vi "总磷总氮通讯.vi"() -> ()   [LabVIEW 2016, in "斯坦道氨氮.lvlib"]
uses:
  <vilib>/Utility/config.llb/NI_LVConfig.lvlib
  <vilib>/Plasmionique/MB Master/MB_Master/MB_Master.lvclass
  <vilib>/Plasmionique/MB Master/MB Master.lvlib
  <vilib>/ptbypt/NI_PtbyPt.lvlib
  <vilib>/Plasmionique/MB Master/MB_Master_Serial/MB_Master_Serial.lvclass
  <vilib>/Plasmionique/MB Master/MB_Master_TCP/MB_Master_TCP.lvclass
  <vilib>/Utility/config.llb/Write Key (Boolean).vi
  <vilib>/Utility/config.llb/Write Key (String).vi
  C:/Program Files (x86)/National Instruments/LabVIEW 2016/vi.lib/Plasmionique/MB Master/MB_Master/MB_Master.lvclass
panel:
  out "启用":bool=TRUE
  out "氨氮状态告警区":u16[](array[numeric])
  out "氨氮测量数据区":u16[](array[numeric])
  out "COD测量数据区":u16[](array[numeric])
  out "COD状态告警区":u16[](array[numeric])
  out "总氮测量数据区":u16[](array[numeric])
  out "总氮状态告警区":u16[](array[numeric])
  out "总磷状态告警区":u16[](array[numeric])
  out "总磷测量数据区":u16[](array[numeric])
  out "状态告警区":T1 {"告警代码" items=["无告警", "缺试剂告警", "缺水样告警", "缺蒸馏水告警", "缺标液告警", "仪表漏液告警", "标定异常告警", "超量程告警", "加热异常", "低试剂预警", "超上限告警", "超下限告警", "仪表内部其他异常", "滴定异常告警", "电极异常告警", "量程切换告警", "参数设置告警", "PH电极电位异常", "电导率电极异常", "浊度光度异常", "溶解氧电极异常", "溶解氧光强异常", "温度异常告警", "PH异常告警", "溶解氧异常告警", "电导率异常告警", "浊度异常告警", "叶绿素异常告警", "藻密度异常告警", "蓝绿藻异常告警", "ORP异常告警", "氨氮异常告警", "清洁刷异常告警", "SD卡异常告警", "蓝牙异常告警", "Wifi异常告警", "流程异常告警"]; "故障代码" items=["无故障", "电机故障", "温度故障", "通讯故障", "滴定故障"]}
  out "测量数据区":T2 {"单位" items=["ug/L", "mg/L", "ppm", "mg/m3", "cm", "ppb", "ug/m3", "%", "nmol/mol", "umol/mol", "MPN/L", "MPN/100ml", "ng/m3", "NTU", "无量纲", "ms/cm", "us/cm", "℃", "mV", "万个/L"]}
  out "status":bool
  out "关键参数区":T3
  in  "读关键参数区":bool
  in  "读状态告警区":bool
  in  "读测量数据区":bool
  in  "站号":u16(ring) items=["总磷"=1, "氨氮"=3]
  in  "停止":bool
  in  "启动":bool
  in  "控制命令":u16(ring) items=["启动测量"=1, "标样核查"=2, "零点核查"=3, "跨度核查"=4, "空白测试"=5, "平行样测试"=6, "加标回收"=7, "空白校准"=8, "标样校准"=9, "初始化（清洗）"=10, "停止测试"=11, "仪器重启"=12, "校时"=13, "模式设置"=14, "测量间隔设置"=15]
  in  "控制命令参数":u16[](array[numeric]) format="%04xH"
  in  "VISA Resource":refnum<visa-resource-name>
  in  "启用模块":bool
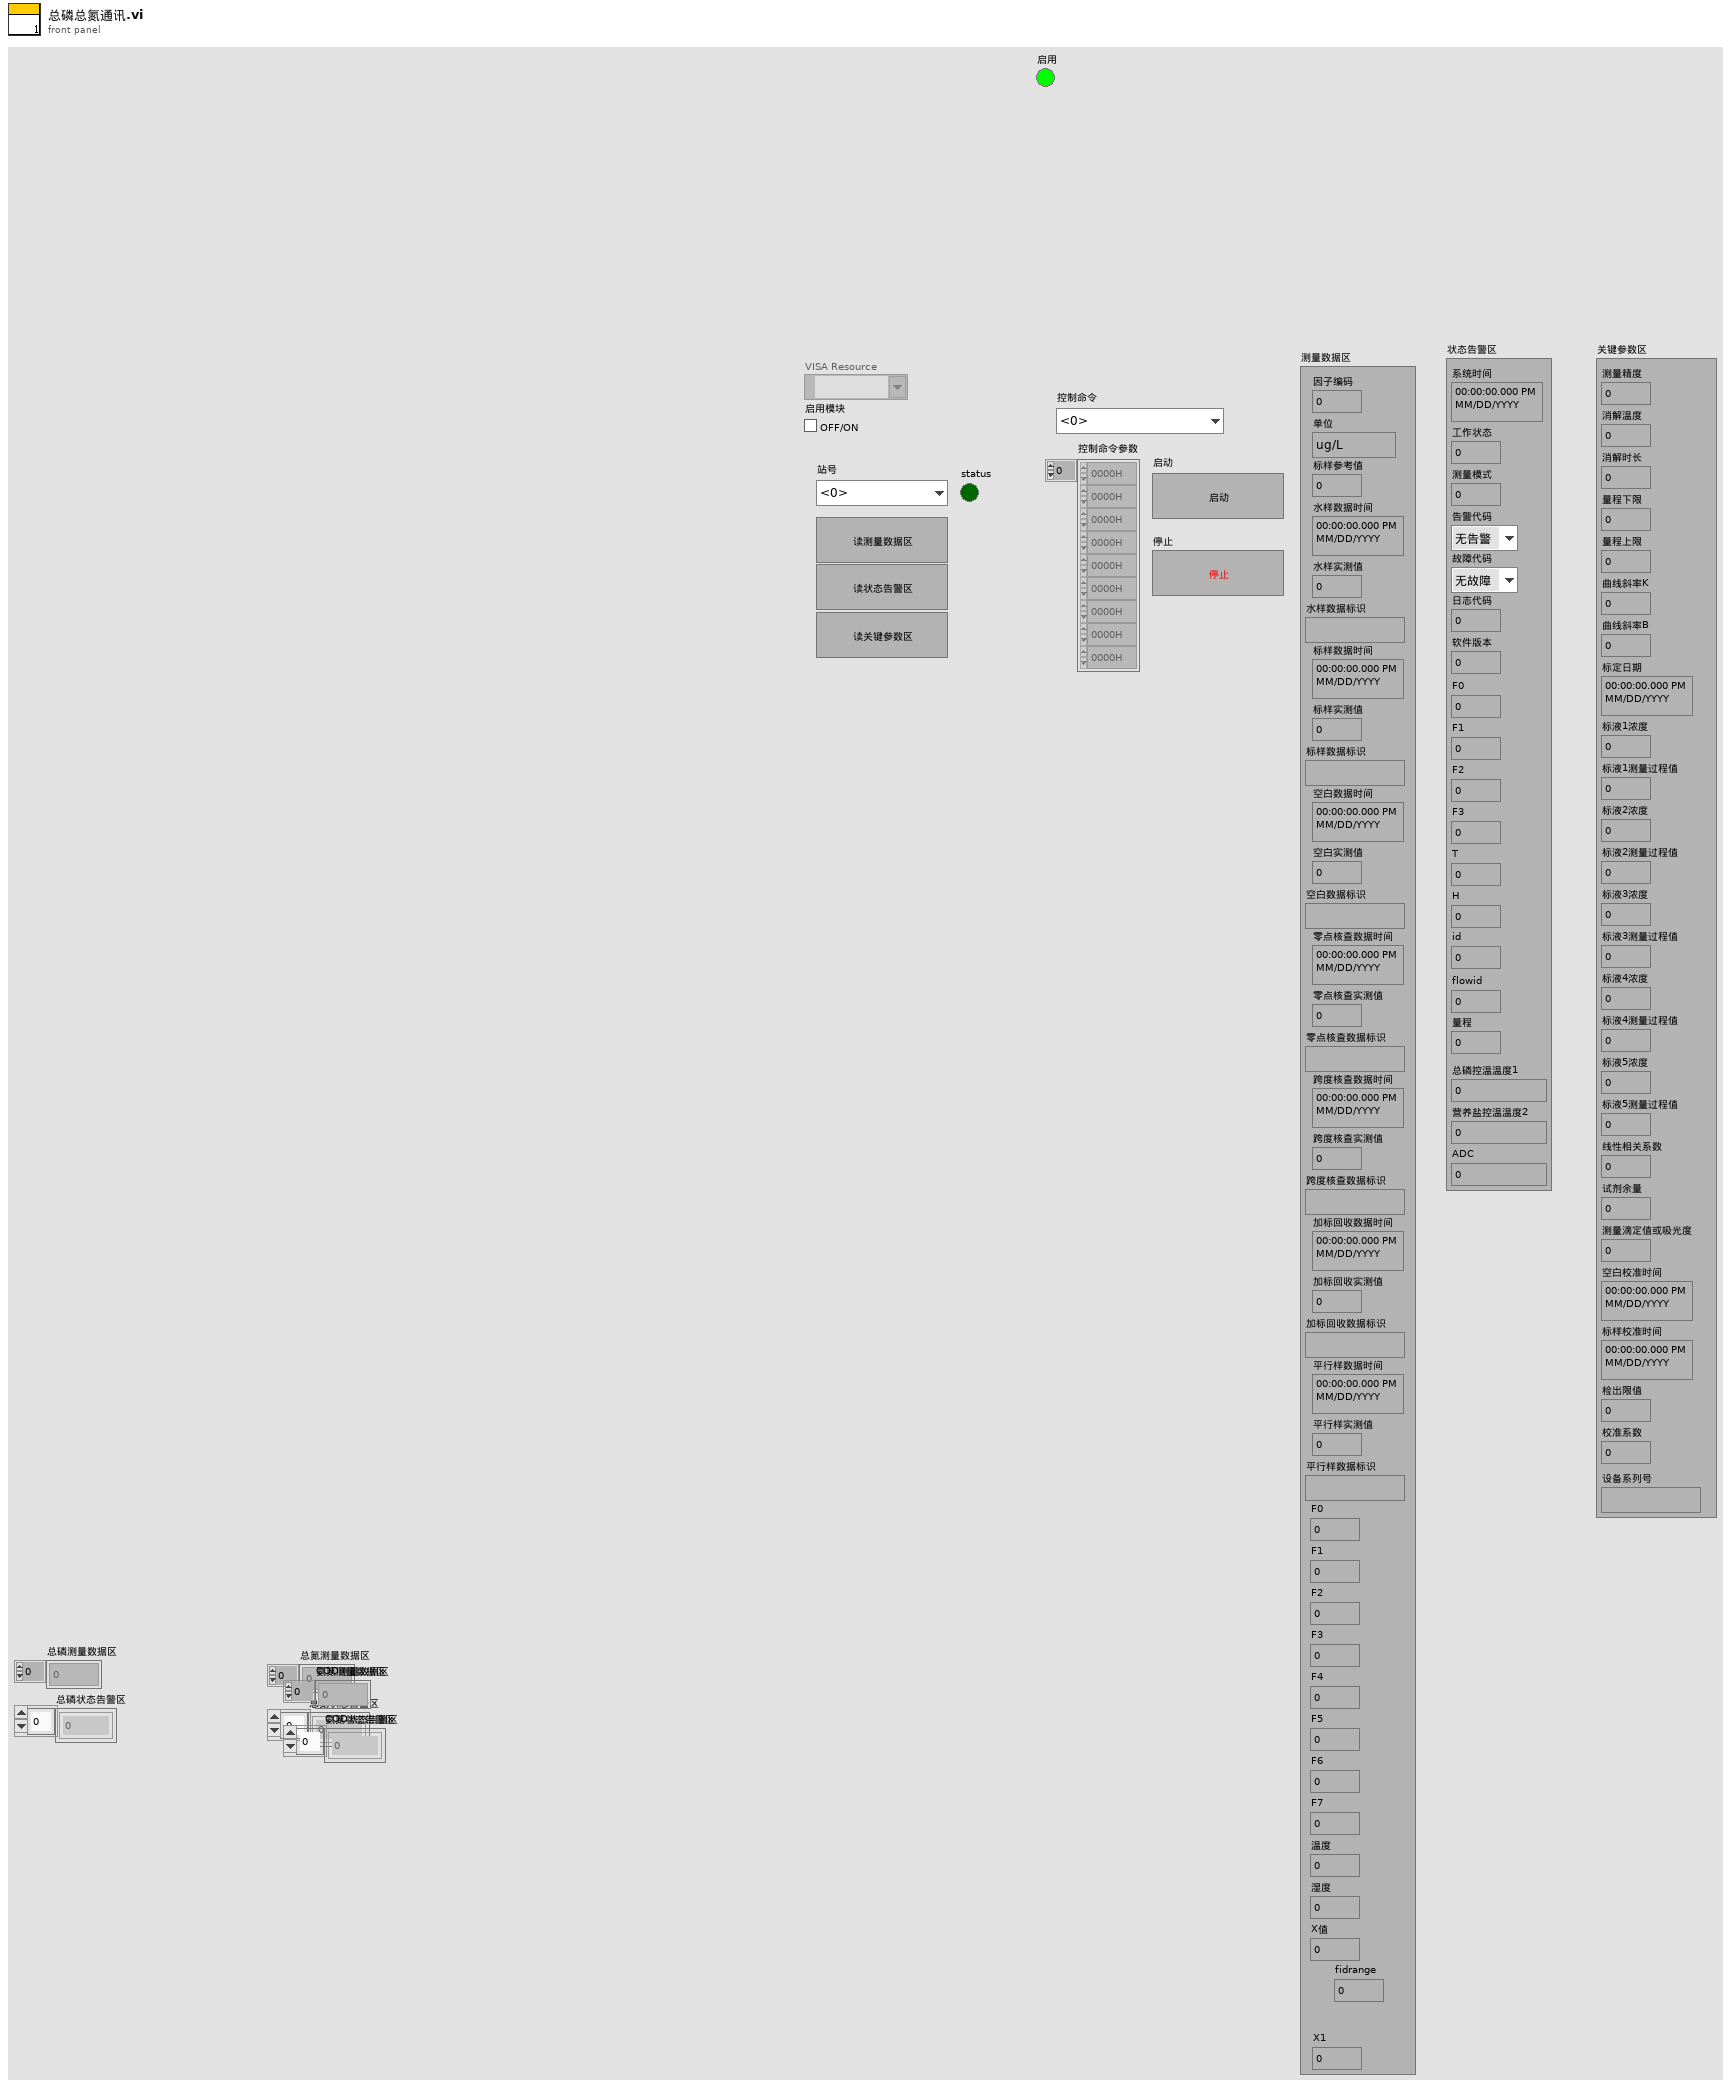
[diagram p1: front panel]
types:
  T1 = cluster{"系统时间":timestamp, "工作状态":u16, "测量模式":u16, "告警代码":u16, "故障代码":u16, "日志代码":u16, "软件版本":u16, "F0":sgl, "F1":sgl, "F2":sgl, "F3":sgl, "T":sgl, "H":sgl, "id":u16, "flowid":u16, "量程":u16, "总磷控温温度1":sgl, "营养盐控温温度2":sgl, "ADC":sgl}
  T2 = cluster{"因子编码":u32, "单位":u16, "标样参考值":sgl, "水样数据时间":timestamp, "水样实测值":sgl, "水样数据标识":string, "标样数据时间":timestamp, "标样实测值":sgl, "标样数据标识":string, "空白数据时间":timestamp, "空白实测值":sgl, "空白数据标识":string, "零点核查数据时间":timestamp, "零点核查实测值":sgl, "零点核查数据标识":string, "跨度核查数据时间":timestamp, "跨度核查实测值":sgl, "跨度核查数据标识":string, "加标回收数据时间":timestamp, "加标回收实测值":sgl, "加标回收数据标识":string, "平行样数据时间":timestamp, "平行样实测值":sgl, "平行样数据标识":string, "F0":sgl, "F1":sgl, "F2":sgl, "F3":sgl, "F4":sgl, "F5":sgl, "F6":sgl, "F7":sgl, "温度":sgl, "湿度":sgl, "X值":sgl, "fidrange":u16, "X1":sgl}
  T3 = cluster{"测量精度":u16, "消解温度":u16, "消解时长":u16, "量程下限":sgl, "量程上限":sgl, "曲线斜率K":sgl, "曲线斜率B":sgl, "标定日期":timestamp, "标液1浓度":sgl, "标液1测量过程值":sgl, "标液2浓度":sgl, "标液2测量过程值":sgl, "标液3浓度":sgl, "标液3测量过程值":sgl, "标液4浓度":sgl, "标液4测量过程值":sgl, "标液5浓度":sgl, "标液5测量过程值":sgl, "线性相关系数":sgl, "试剂余量":u32, "测量滴定值或吸光度":sgl, "空白校准时间":timestamp, "标样校准时间":timestamp, "检出限值":sgl, "校准系数":sgl, "设备系列号":string}
  T4 = cluster{"系统时间":timestamp, "工作状态":u16, "测量模式":enum16{"待机", "连续模式", "周期模式", "定点模式", "受控模式", "手动模式"}, "告警代码":u16, "故障代码":u16, "日志代码":u16, "软件版本":u16, "F0":sgl, "F1":sgl, "F2":sgl, "F3":sgl, "T":sgl, "H":sgl, "id":u16, "flowid":u16, "量程":u16, "总磷控温温度1":sgl, "营养盐控温温度2":sgl, "ADC":sgl}
  T5 = cluster{"因子编码":u32, "单位":u16, "标样参考值":sgl, "水样数据时间":timestamp, "水样实测值":sgl, "水样数据标识":string, "标样数据时间":timestamp, "标样实测值":sgl, "标样数据标识":string, "空白数据时间":timestamp, "空白实测值":sgl, "空白数据标识":string, "零点核查数据时间":timestamp, "零点核查实测值":sgl, "零点核查数据标识":string, "跨度核查数据时间":timestamp, "跨度核查实测值":sgl, "跨度核查数据标识":string, "加标回收数据时间":timestamp, "加标回收实测值":sgl, "加标回收数据标识":string, "平行样数据时间":timestamp, "平行样实测值":sgl, "平行样数据标识":string, "F0":sgl, "F1":sgl, "F2":sgl, "F3":sgl, "F4":sgl, "F5":sgl, "F6":sgl, "F7":sgl, "温度":sgl, "湿度":sgl, "X值":sgl, "fidrange":u16, "X1值":sgl}
  T6 = cluster{"测量精度":u16, "消解温度":u16, "消解时长":u16, "量程下限":sgl, "量程上限":sgl, "曲线斜率K":sgl, "曲线斜率B":sgl, "标定日期":timestamp, "标液1浓度":sgl, "标液1测量过程值":sgl, "标液2浓度":sgl, "标液2测量过程值":sgl, "标液3浓度":sgl, "标液3测量过程值":sgl, "标液4浓度":sgl, "标液4测量过程值":sgl, "标液5浓度":sgl, "标液5测量过程值":sgl, "线性相关系数":sgl, "试剂余量":u32, "测量滴定值或吸光度":sgl, "空白校准时间":timestamp, "标样校准时间":timestamp, "检出限值":sgl, "校准系数":sgl, "设备系列号":string}[]
  T7 = cluster{"系统时间":timestamp, "工作状态":u16, "测量模式":enum16{"待机", "连续模式", "周期模式", "定点模式", "受控模式", "手动模式"}, "告警代码":u16, "故障代码":u16, "日志代码":u16, "软件版本":u16, "F0":sgl, "F1":sgl, "F2":sgl, "F3":sgl, "T":sgl, "H":sgl, "id":u16, "flowid":u16, "量程":u16, "总磷控温温度1":sgl, "营养盐控温温度2":sgl, "ADC":sgl}[]
  T8 = cluster{"因子编码":u32, "单位":u16, "标样参考值":sgl, "水样数据时间":timestamp, "水样实测值":sgl, "水样数据标识":string, "标样数据时间":timestamp, "标样实测值":sgl, "标样数据标识":string, "空白数据时间":timestamp, "空白实测值":sgl, "空白数据标识":string, "零点核查数据时间":timestamp, "零点核查实测值":sgl, "零点核查数据标识":string, "跨度核查数据时间":timestamp, "跨度核查实测值":sgl, "跨度核查数据标识":string, "加标回收数据时间":timestamp, "加标回收实测值":sgl, "加标回收数据标识":string, "平行样数据时间":timestamp, "平行样实测值":sgl, "平行样数据标识":string, "F0":sgl, "F1":sgl, "F2":sgl, "F3":sgl, "F4":sgl, "F5":sgl, "F6":sgl, "F7":sgl, "温度":sgl, "湿度":sgl, "X值":sgl, "fidrange":u16, "X1值":sgl}[]
  T9 = typedef "CODCr交互.ctl" = cluster{"状态告警区":cluster{"系统时间":timestamp, "工作状态":u16, "测量模式":enum16{"待机", "连续模式", "周期模式", "定点模式", "受控模式", "手动模式"}, "告警代码":u16, "故障代码":u16, "日志代码":u16, "软件版本":u16, "F0":sgl, "F1":sgl, "F2":sgl, "F3":sgl, "T":sgl, "H":sgl, "id":u16, "flowid":u16, "量程":u16, "总磷控温温度1":sgl, "营养盐控温温度2":sgl, "ADC":sgl}, "平台试剂余量百分比":sgl, "关键参数":cluster{"测量量程":dbl, "测量精度":dbl, "测量间隔":dbl, "消解温度":dbl, "消解时长":dbl, "空白校准时间":timestamp, "曲线截距":dbl, "曲线斜率":dbl, "测量检出限":dbl, "测量信号值":dbl, "线性相关系数":dbl, "二次多项式系数":dbl, "标样校准时间":timestamp, "稀释倍数":dbl, "三项式系数":dbl, "空白标定系数":dbl, "量程系数":dbl, "F0/ORPA":dbl, "F1/ORPB":dbl, "F2/ORPK":dbl, "F3":dbl, "F4":dbl, "F5":dbl, "F6":dbl, "F7":dbl, "X0/滴定数":dbl, "量程":dbl}, "关键参数改变":bool, "校准信息":cluster{"低标液1浓度":dbl, "低标液1信号值":dbl, "低标液1启用":u16, "低标液2浓度":dbl, "低标液2信号值":dbl, "低标液2启用":u16, "低标液3浓度":dbl, "低标液3信号值":dbl, "低标液3启用":u16, "低标液4浓度":dbl, "低标液4信号值":dbl, "低标液4启用":u16, "低标液5浓度":dbl, "低标液5信号值":dbl, "低标液5启用":u16, "高标液1浓度":dbl, "高标液1信号值":dbl, "高标液1启用":u16, "高标液2浓度":dbl, "高标液2信号值":dbl, "高标液2启用":u16, "高标液3浓度":dbl, "高标液3信号值":dbl, "高标液3启用":u16, "高标液4浓度":dbl, "高标液4信号值":dbl, "高标液4启用":u16, "高标液5浓度":dbl, "高标液5信号值":dbl, "高标液5启用":u16}, "校准信息改变":bool}
  T10 = typedef "总磷交互.ctl" = cluster{"状态告警区":cluster{"系统时间":timestamp, "工作状态":u16, "测量模式":enum16{"待机", "连续模式", "周期模式", "定点模式", "受控模式", "手动模式"}, "告警代码":u16, "故障代码":u16, "日志代码":u16, "软件版本":u16, "F0":sgl, "F1":sgl, "F2":sgl, "F3":sgl, "T":sgl, "H":sgl, "id":u16, "flowid":u16, "量程":u16, "总磷控温温度1":sgl, "营养盐控温温度2":sgl, "ADC":sgl}, "平台试剂余量百分比":sgl, "关键参数":cluster{"测量量程":dbl, "测量精度":dbl, "测量间隔":dbl, "消解温度":dbl, "消解时长":dbl, "空白校准时间":timestamp, "曲线截距":dbl, "曲线斜率":dbl, "测量检出限":dbl, "测量信号值":dbl, "线性相关系数":dbl, "二次多项式系数":dbl, "标样校准时间":timestamp, "稀释倍数":dbl, "三项式系数":dbl, "空白标定系数":dbl, "量程系数":dbl, "F0/ORPA":dbl, "F1/ORPB":dbl, "F2/ORPK":dbl, "F3":dbl, "F4":dbl, "F5":dbl, "F6":dbl, "F7":dbl, "X0/滴定数":dbl, "量程":dbl}, "关键参数改变":bool, "校准信息":cluster{"低标液1浓度":dbl, "低标液1信号值":dbl, "低标液1启用":u16, "低标液2浓度":dbl, "低标液2信号值":dbl, "低标液2启用":u16, "低标液3浓度":dbl, "低标液3信号值":dbl, "低标液3启用":u16, "低标液4浓度":dbl, "低标液4信号值":dbl, "低标液4启用":u16, "低标液5浓度":dbl, "低标液5信号值":dbl, "低标液5启用":u16, "高标液1浓度":dbl, "高标液1信号值":dbl, "高标液1启用":u16, "高标液2浓度":dbl, "高标液2信号值":dbl, "高标液2启用":u16, "高标液3浓度":dbl, "高标液3信号值":dbl, "高标液3启用":u16, "高标液4浓度":dbl, "高标液4信号值":dbl, "高标液4启用":u16, "高标液5浓度":dbl, "高标液5信号值":dbl, "高标液5启用":u16}, "校准信息改变":bool}
  T11 = typedef "总氮交互.ctl" = cluster{"状态告警区":cluster{"系统时间":timestamp, "工作状态":u16, "测量模式":enum16{"待机", "连续模式", "周期模式", "定点模式", "受控模式", "手动模式"}, "告警代码":u16, "故障代码":u16, "日志代码":u16, "软件版本":u16, "F0":sgl, "F1":sgl, "F2":sgl, "F3":sgl, "T":sgl, "H":sgl, "id":u16, "flowid":u16, "量程":u16, "总磷控温温度1":sgl, "营养盐控温温度2":sgl, "ADC":sgl}, "平台试剂余量百分比":sgl, "关键参数":cluster{"测量量程":dbl, "测量精度":dbl, "测量间隔":dbl, "消解温度":dbl, "消解时长":dbl, "空白校准时间":timestamp, "曲线截距":dbl, "曲线斜率":dbl, "测量检出限":dbl, "测量信号值":dbl, "线性相关系数":dbl, "二次多项式系数":dbl, "标样校准时间":timestamp, "稀释倍数":dbl, "三项式系数":dbl, "空白标定系数":dbl, "量程系数":dbl, "F0/ORPA":dbl, "F1/ORPB":dbl, "F2/ORPK":dbl, "F3":dbl, "F4":dbl, "F5":dbl, "F6":dbl, "F7":dbl, "X0/滴定数":dbl, "量程":dbl}, "关键参数改变":bool, "校准信息":cluster{"低标液1浓度":dbl, "低标液1信号值":dbl, "低标液1启用":u16, "低标液2浓度":dbl, "低标液2信号值":dbl, "低标液2启用":u16, "低标液3浓度":dbl, "低标液3信号值":dbl, "低标液3启用":u16, "低标液4浓度":dbl, "低标液4信号值":dbl, "低标液4启用":u16, "低标液5浓度":dbl, "低标液5信号值":dbl, "低标液5启用":u16, "高标液1浓度":dbl, "高标液1信号值":dbl, "高标液1启用":u16, "高标液2浓度":dbl, "高标液2信号值":dbl, "高标液2启用":u16, "高标液3浓度":dbl, "高标液3信号值":dbl, "高标液3启用":u16, "高标液4浓度":dbl, "高标液4信号值":dbl, "高标液4启用":u16, "高标液5浓度":dbl, "高标液5信号值":dbl, "高标液5启用":u16}, "校准信息改变":bool}
  T12 = typedef "氨氮交互.ctl" = cluster{"状态告警区":cluster{"系统时间":timestamp, "工作状态":u16, "测量模式":enum16{"待机", "连续模式", "周期模式", "定点模式", "受控模式", "手动模式"}, "告警代码":u16, "故障代码":u16, "日志代码":u16, "软件版本":u16, "F0":sgl, "F1":sgl, "F2":sgl, "F3":sgl, "T":sgl, "H":sgl, "id":u16, "flowid":u16, "量程":u16, "总磷控温温度1":sgl, "营养盐控温温度2":sgl, "ADC":sgl}, "平台试剂余量百分比":sgl, "关键参数":cluster{"测量量程":dbl, "测量精度":dbl, "测量间隔":dbl, "消解温度":dbl, "消解时长":dbl, "空白校准时间":timestamp, "曲线截距":dbl, "曲线斜率":dbl, "测量检出限":dbl, "测量信号值":dbl, "线性相关系数":dbl, "二次多项式系数":dbl, "标样校准时间":timestamp, "稀释倍数":dbl, "三项式系数":dbl, "空白标定系数":dbl, "量程系数":dbl, "F0/ORPA":dbl, "F1/ORPB":dbl, "F2/ORPK":dbl, "F3":dbl, "F4":dbl, "F5":dbl, "F6":dbl, "F7":dbl, "X0/滴定数":dbl, "量程":dbl}, "关键参数改变":bool, "校准信息":cluster{"低标液1浓度":dbl, "低标液1信号值":dbl, "低标液1启用":u16, "低标液2浓度":dbl, "低标液2信号值":dbl, "低标液2启用":u16, "低标液3浓度":dbl, "低标液3信号值":dbl, "低标液3启用":u16, "低标液4浓度":dbl, "低标液4信号值":dbl, "低标液4启用":u16, "低标液5浓度":dbl, "低标液5信号值":dbl, "低标液5启用":u16, "高标液1浓度":dbl, "高标液1信号值":dbl, "高标液1启用":u16, "高标液2浓度":dbl, "高标液2信号值":dbl, "高标液2启用":u16, "高标液3浓度":dbl, "高标液3信号值":dbl, "高标液3启用":u16, "高标液4浓度":dbl, "高标液4信号值":dbl, "高标液4启用":u16, "高标液5浓度":dbl, "高标液5信号值":dbl, "高标液5启用":u16}, "校准信息改变":bool}
  T13 = typedef "NI_LVConfig.lvlib/Config Data RefNum.ctl" = refnum<k1>
  T14 = enum8{"Enabled", "Disabled", "Disabled and Grayed Out"}
  T15 = typedef "报警信息字段定义.ctl" = cluster{"时间":timestamp, "参数":string, "报警信息":string, "备注":string, "code":u64, "platform_alarm_code":string, "报警标识":enum16{"产生", "消除"}}
  T16 = cluster{"baud rate (bps)":u32, "stop bits":u16, "parity":u16, "flow control":u16, "timeout":u32, "retries":i32}
  T17 = cluster{"测量量程":dbl, "测量精度":dbl, "测量间隔":dbl, "消解温度":dbl, "消解时长":dbl, "空白校准时间":timestamp, "曲线截距":dbl, "曲线斜率":dbl, "测量检出限":dbl, "测量信号值":dbl, "线性相关系数":dbl, "二次多项式系数":dbl, "标样校准时间":timestamp, "稀释倍数":dbl, "三项式系数":dbl, "空白标定系数":dbl, "量程系数":dbl, "F0/ORPA":dbl, "F1/ORPB":dbl, "F2/ORPK":dbl, "F3":dbl, "F4":dbl, "F5":dbl, "F6":dbl, "F7":dbl, "X0/滴定数":dbl, "量程":dbl}
  T18 = typedef "斯坦道氨氮.lvlib/关键参数.ctl" = cluster{"测量量程":sgl, "测量检出限":sgl, "测量精度":sgl, "测量间隔":sgl, "消解温度":sgl, "消解时长":sgl, "三项式系数":sgl, "二次多项式系数":sgl, "曲线斜率":sgl, "曲线截距":sgl, "线性相关系数":sgl, "空白校准时间":timestamp, "标样校准时间":timestamp, "测量信号值":sgl, "稀释倍数":sgl, "空白标定系数":sgl, "量程系数":sgl}
  T19 = cluster{"低标液1浓度":dbl, "低标液1信号值":dbl, "低标液1启用":u16, "低标液2浓度":dbl, "低标液2信号值":dbl, "低标液2启用":u16, "低标液3浓度":dbl, "低标液3信号值":dbl, "低标液3启用":u16, "低标液4浓度":dbl, "低标液4信号值":dbl, "低标液4启用":u16, "低标液5浓度":dbl, "低标液5信号值":dbl, "低标液5启用":u16, "高标液1浓度":dbl, "高标液1信号值":dbl, "高标液1启用":u16, "高标液2浓度":dbl, "高标液2信号值":dbl, "高标液2启用":u16, "高标液3浓度":dbl, "高标液3信号值":dbl, "高标液3启用":u16, "高标液4浓度":dbl, "高标液4信号值":dbl, "高标液4启用":u16, "高标液5浓度":dbl, "高标液5信号值":dbl, "高标液5启用":u16, "低斜率":dbl, "低截距":dbl, "低二次多项式系数":dbl, "低线性相关系数":dbl, "高斜率":dbl, "高截距":dbl, "高二次多项式系数":dbl, "高线性相关系数":dbl}
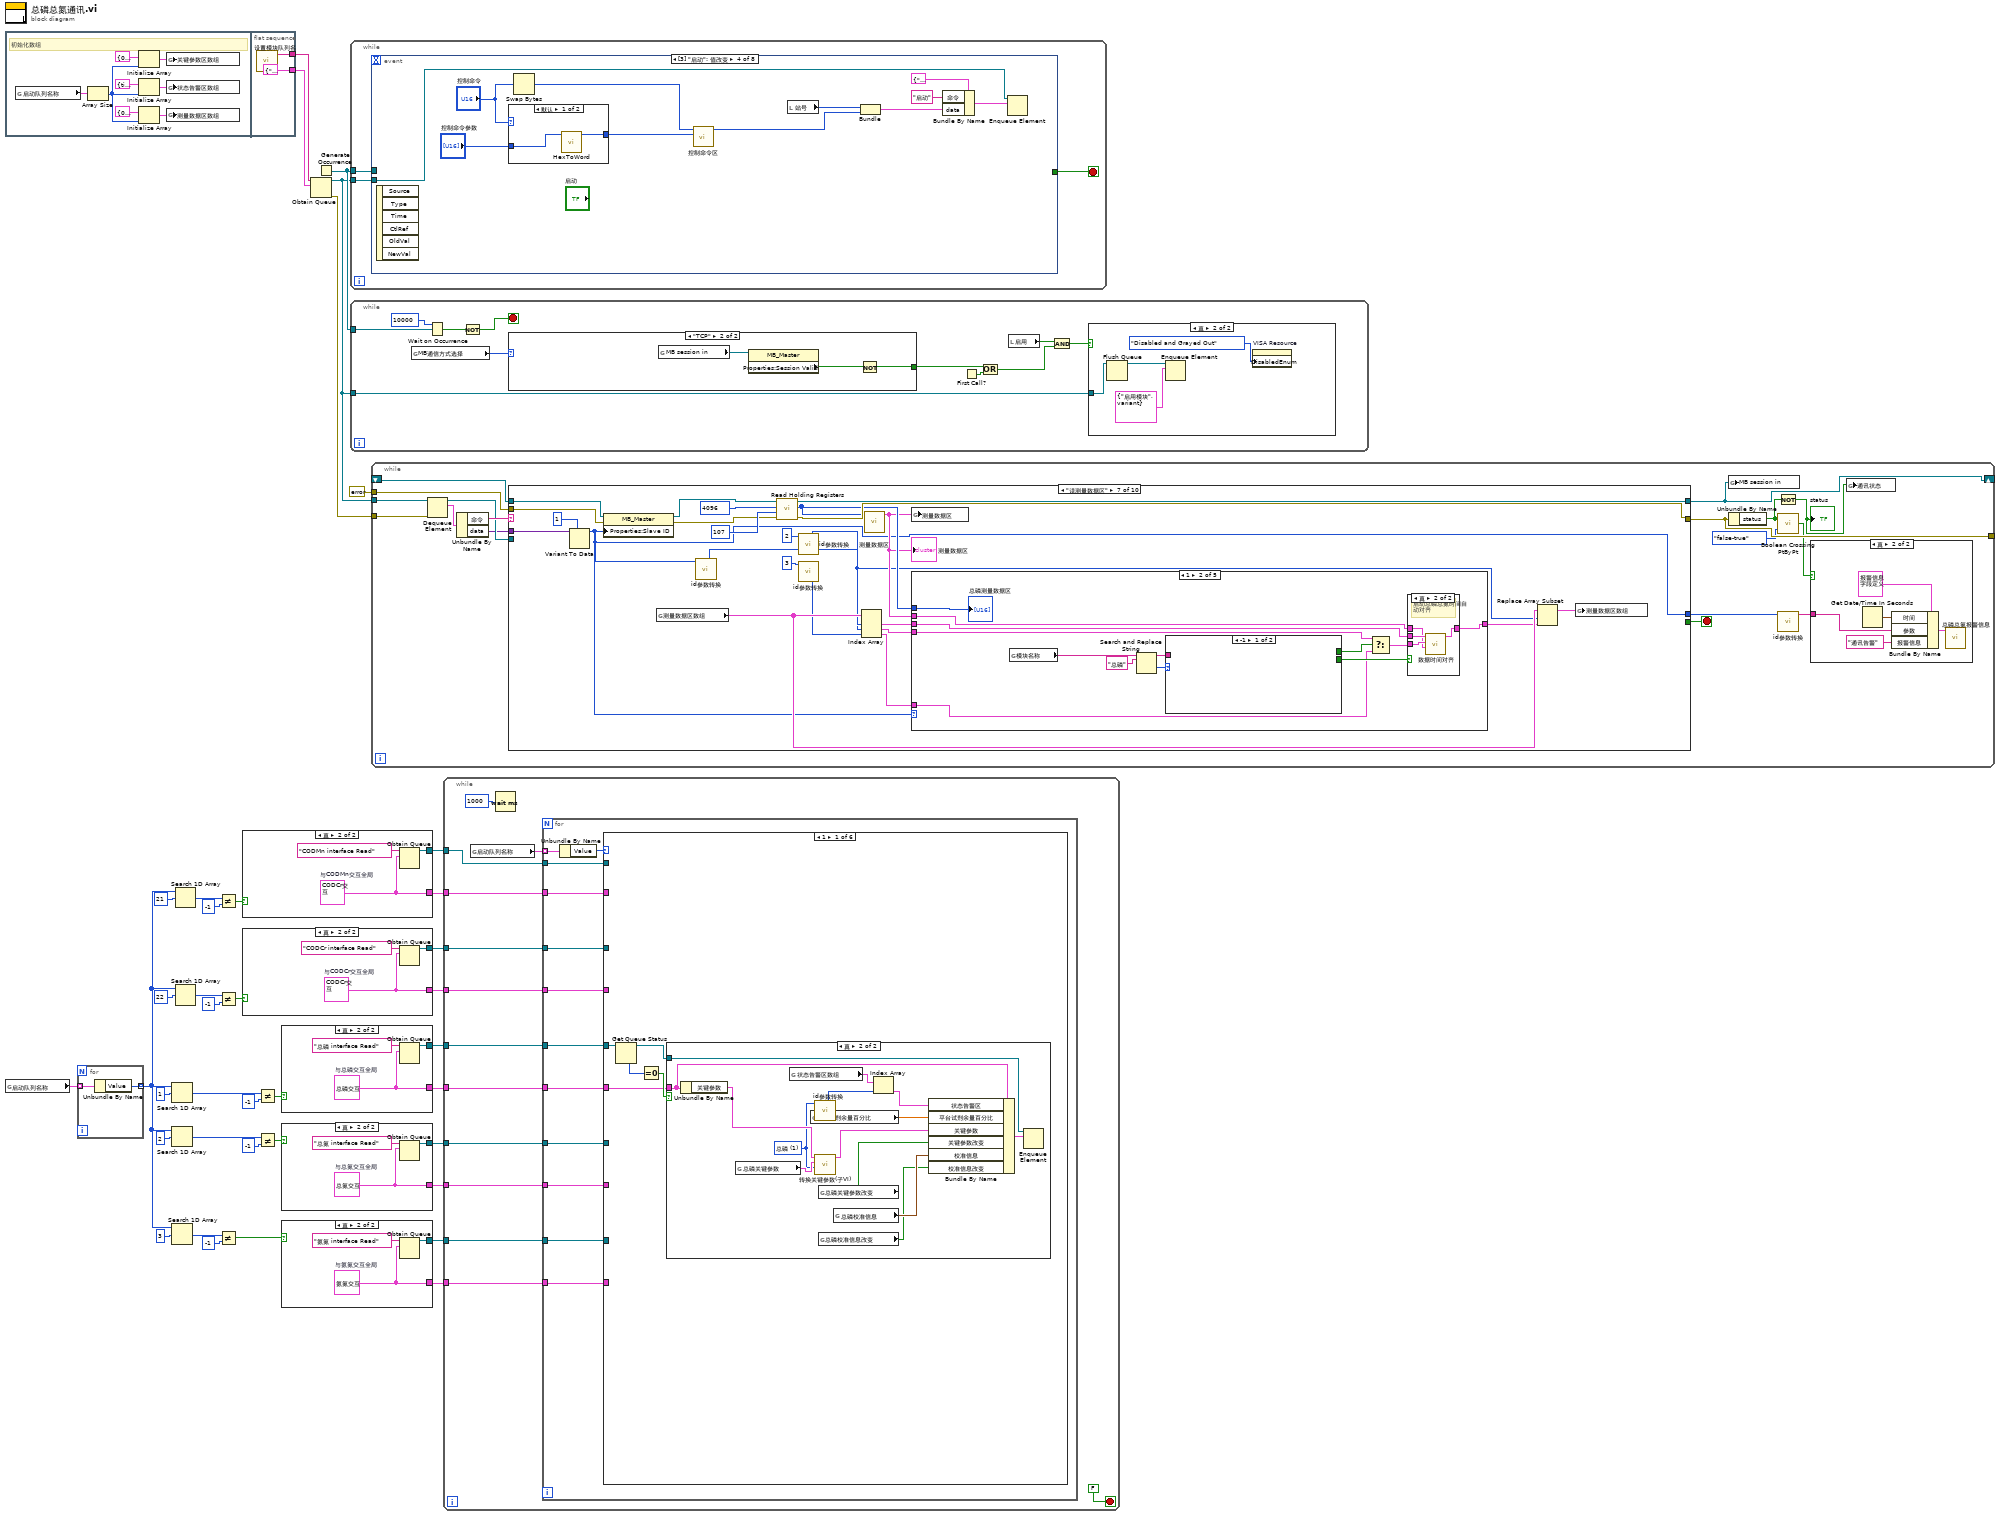
[diagram p0: block diagram]
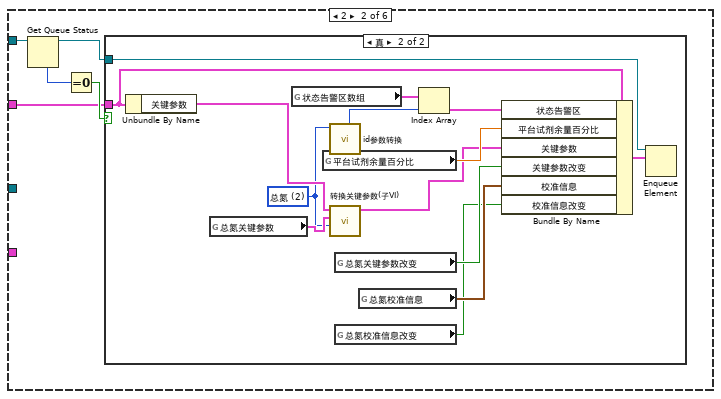
[diagram p8: hidden frame]
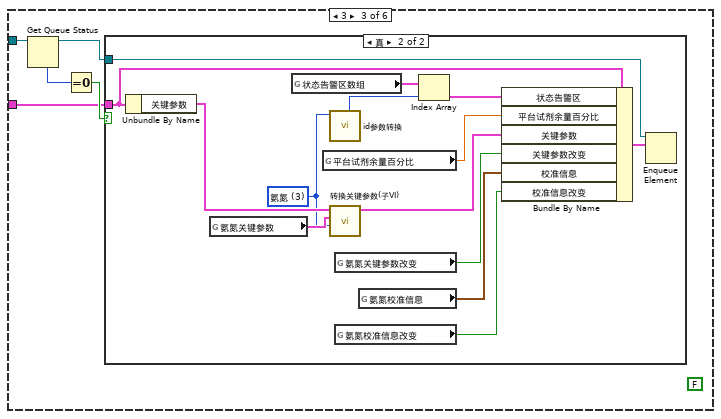
[diagram p10: hidden frame]
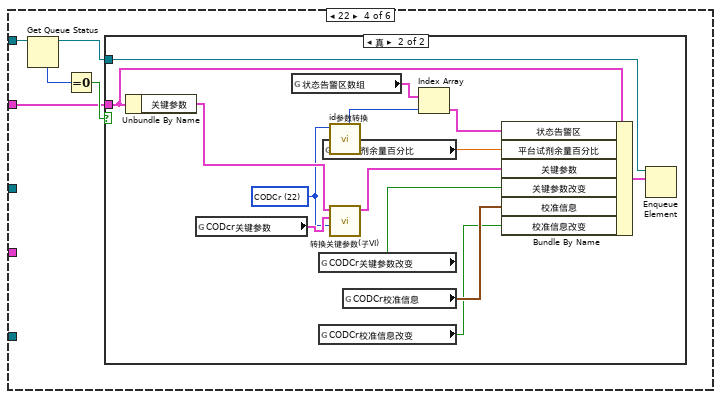
[diagram p12: hidden frame]
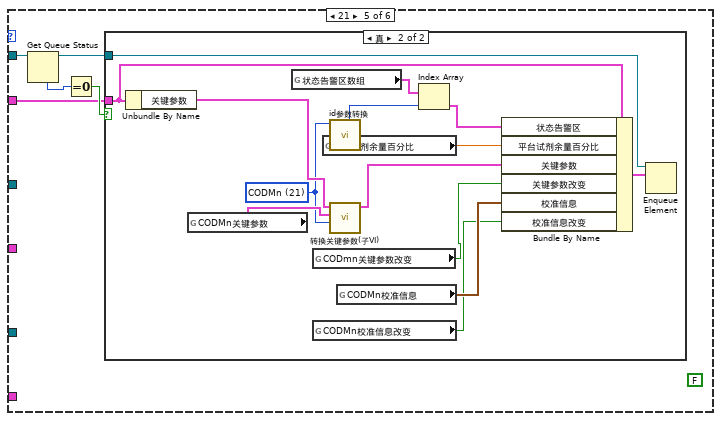
[diagram p14: hidden frame]
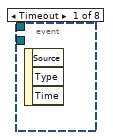
[diagram p19: hidden frame]
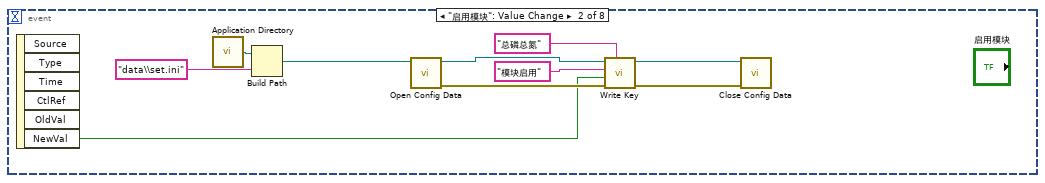
[diagram p20: hidden frame]
diagram:
  n1 = flat-sequence {
    tunnel: [cluster{"命令":string, "data":variant} {"命令"="", "data"=variant}] -> w38
    tunnel: [w47] -> w33
    frame #0 {
      # "初始化数组"
      n2 = global read "model config var.vi" "启动队列名称"() -> (w40:cluster{"String":string, "Value":u16}[])
      n3 = Array Size(array=w40) -> (size(s)=w39:i32)
      n4 = Initialize Array(T3 {"测量精度"=0, "消解温度"=0, "消解时长"=0, "量程下限"=0.0, "量程上限"=0.0, "曲线斜率K"=0.0, "曲线斜率B"=0.0, "标定日期"=timestamp(0 s since 1904-01-01), "标液1浓度"=0.0, "标液1测量过程值"=0.0, "标液2浓度"=0.0, "标液2测量过程值"=0.0, "标液3浓度"=0.0, "标液3测量过程值"=0.0, "标液4浓度"=0.0, "标液4测量过程值"=0.0, "标液5浓度"=0.0, "标液5测量过程值"=0.0, "线性相关系数"=0.0, "试剂余量"=0, "测量滴定值或吸光度"=0.0, "空白校准时间"=timestamp(0 s since 1904-01-01), "标样校准时间"=timestamp(0 s since 1904-01-01), "检出限值"=0.0, "校准系数"=0.0, "设备系列号"=""} ("关键参数区"), w39) -> (w44:T6)
      n5 = Initialize Array(T4 {"系统时间"=timestamp(0 s since 1904-01-01), "工作状态"=0, "测量模式"=enum."待机", "告警代码"=0, "故障代码"=0, "日志代码"=0, "软件版本"=0, "F0"=0.0, "F1"=0.0, "F2"=0.0, "F3"=0.0, "T"=0.0, "H"=0.0, "id"=0, "flowid"=0, "量程"=0, "总磷控温温度1"=0.0, "营养盐控温温度2"=0.0, "ADC"=0.0} ("状态告警区"), w39) -> (w43:T7)
      n6 = Initialize Array(T5 {"因子编码"=0, "单位"=0, "标样参考值"=0.0, "水样数据时间"=timestamp(0 s since 1904-01-01), "水样实测值"=0.0, "水样数据标识"="", "标样数据时间"=timestamp(0 s since 1904-01-01), "标样实测值"=0.0, "标样数据标识"="", "空白数据时间"=timestamp(0 s since 1904-01-01), "空白实测值"=0.0, "空白数据标识"="", "零点核查数据时间"=timestamp(0 s since 1904-01-01), "零点核查实测值"=0.0, "零点核查数据标识"="", "跨度核查数据时间"=timestamp(0 s since 1904-01-01), "跨度核查实测值"=0.0, "跨度核查数据标识"="", "加标回收数据时间"=timestamp(0 s since 1904-01-01), "加标回收实测值"=0.0, "加标回收数据标识"="", "平行样数据时间"=timestamp(0 s since 1904-01-01), "平行样实测值"=0.0, "平行样数据标识"="", "F0"=0.0, "F1"=0.0, "F2"=0.0, "F3"=0.0, "F4"=0.0, "F5"=0.0, "F6"=0.0, "F7"=0.0, "温度"=0.0, "湿度"=0.0, "X值"=0.0, "fidrange"=0, "X1值"=0.0} ("测量数据区"), w39) -> (w46:T8)
      n7 = global write "VAR总磷总氮全局变量.vi" "关键参数区数组"(w44) -> ()
      n8 = global write "VAR总磷总氮全局变量.vi" "状态告警区数组"(w43) -> ()
      n9 = global write "VAR总磷总氮全局变量.vi" "测量数据区数组"(w46) -> ()
    }
    frame #1 {
      n10 = call "设置模块队列名.vi"() -> ("Msg"=w47:string)  [unwired: 5 in]
    }
  }
  n11 = global read "model config var.vi" "启动队列名称"() -> (w22:cluster{"String":string, "Value":u16}[])
  n12 = for {
    tunnel: w22 -> [w50] mode=indexing
    tunnel: [w49] -> w2 mode=indexing
    n13 = Unbundle By Name(w50) -> ("Value"=w49:u16)
  }
  n14 = Search 1D Array(1D array=w2, element=u16 1 ("元素")) -> (index of element=w12:i32)  [unwired: 1 in]
  n15 = Search 1D Array(1D array=w2, element=u16 2 ("元素")) -> (index of element=w8:i32)  [unwired: 1 in]
  n16 = Search 1D Array(1D array=w2, element=u16 3 ("元素")) -> (index of element=w4:i32)  [unwired: 1 in]
  n17 = Search 1D Array(1D array=w2, element=u16 21 ("元素")) -> (index of element=w20:i32)  [unwired: 1 in]
  n18 = Search 1D Array(1D array=w2, element=u16 22 ("元素")) -> (index of element=w16:i32)  [unwired: 1 in]
  n19 = Not Equal?(x=w20, y=-1) -> (x != y?=w18:bool)
  n20 = Not Equal?(x=w16, y=-1) -> (x != y?=w14:bool)
  n21 = Not Equal?(x=w4, y=-1) -> (x != y?=w1:bool)
  n22 = case shown="真" w18 {
    tunnel: [_ w52] -> w32
    tunnel: [_ w51] -> w31
    frame False {
    }
    frame True {
      w51 = T9 {"状态告警区"={"系统时间"=timestamp(0 s since 1904-01-01), "工作状态"=0, "测量模式"=enum."待机", "告警代码"=0, "故障代码"=0, "日志代码"=0, "软件版本"=0, "F0"=0.0, "F1"=0.0, "F2"=0.0, "F3"=0.0, "T"=0.0, "H"=0.0, "id"=0, "flowid"=0, "量程"=0, "总磷控温温度1"=0.0, "营养盐控温温度2"=0.0, "ADC"=0.0}, "平台试剂余量百分比"=0.0, "关键参数"={"测量量程"=0.0, "测量精度"=0.0, "测量间隔"=0.0, "消解温度"=0.0, "消解时长"=0.0, "空白校准时间"=timestamp(0 s since 1904-01-01), "曲线截距"=0.0, "曲线斜率"=0.0, "测量检出限"=0.0, "测量信号值"=0.0, "线性相关系数"=0.0, "二次多项式系数"=0.0, "标样校准时间"=timestamp(0 s since 1904-01-01), "稀释倍数"=0.0, "三项式系数"=0.0, "空白标定系数"=0.0, "量程系数"=0.0, "F0/ORPA"=0.0, "F1/ORPB"=0.0, "F2/ORPK"=0.0, "F3"=0.0, "F4"=0.0, "F5"=0.0, "F6"=0.0, "F7"=0.0, "X0/滴定数"=0.0, "量程"=0.0}, "关键参数改变"=FALSE, "校准信息"={"低标液1浓度"=0.0, "低标液1信号值"=0.0, "低标液1启用"=0, "低标液2浓度"=0.0, "低标液2信号值"=0.0, "低标液2启用"=0, "低标液3浓度"=0.0, "低标液3信号值"=0.0, "低标液3启用"=0, "低标液4浓度"=0.0, "低标液4信号值"=0.0, "低标液4启用"=0, "低标液5浓度"=0.0, "低标液5信号值"=0.0, "低标液5启用"=0, "高标液1浓度"=0.0, "高标液1信号值"=0.0, "高标液1启用"=0, "高标液2浓度"=0.0, "高标液2信号值"=0.0, "高标液2启用"=0, "高标液3浓度"=0.0, "高标液3信号值"=0.0, "高标液3启用"=0, "高标液4浓度"=0.0, "高标液4信号值"=0.0, "高标液4启用"=0, "高标液5浓度"=0.0, "高标液5信号值"=0.0, "高标液5启用"=0}, "校准信息改变"=FALSE}  # 与CODMn交互全局
      n23 = Obtain Queue(name (unnamed)="CODMn interface Read" ("写入方名称"), element data type=w51) -> (queue out=w52:refnum<queue>)  [unwired: 3 in, 2 out]
    }
  }
  n24 = case shown="真" w14 {
    tunnel: [_ w55] -> w30
    tunnel: [_ w54] -> w29
    frame False {
    }
    frame True {
      w54 = T9 {"状态告警区"={"系统时间"=timestamp(0 s since 1904-01-01), "工作状态"=0, "测量模式"=enum."待机", "告警代码"=0, "故障代码"=0, "日志代码"=0, "软件版本"=0, "F0"=0.0, "F1"=0.0, "F2"=0.0, "F3"=0.0, "T"=0.0, "H"=0.0, "id"=0, "flowid"=0, "量程"=0, "总磷控温温度1"=0.0, "营养盐控温温度2"=0.0, "ADC"=0.0}, "平台试剂余量百分比"=0.0, "关键参数"={"测量量程"=0.0, "测量精度"=0.0, "测量间隔"=0.0, "消解温度"=0.0, "消解时长"=0.0, "空白校准时间"=timestamp(0 s since 1904-01-01), "曲线截距"=0.0, "曲线斜率"=0.0, "测量检出限"=0.0, "测量信号值"=0.0, "线性相关系数"=0.0, "二次多项式系数"=0.0, "标样校准时间"=timestamp(0 s since 1904-01-01), "稀释倍数"=0.0, "三项式系数"=0.0, "空白标定系数"=0.0, "量程系数"=0.0, "F0/ORPA"=0.0, "F1/ORPB"=0.0, "F2/ORPK"=0.0, "F3"=0.0, "F4"=0.0, "F5"=0.0, "F6"=0.0, "F7"=0.0, "X0/滴定数"=0.0, "量程"=0.0}, "关键参数改变"=FALSE, "校准信息"={"低标液1浓度"=0.0, "低标液1信号值"=0.0, "低标液1启用"=0, "低标液2浓度"=0.0, "低标液2信号值"=0.0, "低标液2启用"=0, "低标液3浓度"=0.0, "低标液3信号值"=0.0, "低标液3启用"=0, "低标液4浓度"=0.0, "低标液4信号值"=0.0, "低标液4启用"=0, "低标液5浓度"=0.0, "低标液5信号值"=0.0, "低标液5启用"=0, "高标液1浓度"=0.0, "高标液1信号值"=0.0, "高标液1启用"=0, "高标液2浓度"=0.0, "高标液2信号值"=0.0, "高标液2启用"=0, "高标液3浓度"=0.0, "高标液3信号值"=0.0, "高标液3启用"=0, "高标液4浓度"=0.0, "高标液4信号值"=0.0, "高标液4启用"=0, "高标液5浓度"=0.0, "高标液5信号值"=0.0, "高标液5启用"=0}, "校准信息改变"=FALSE}  # 与CODCr交互全局
      n25 = Obtain Queue(name (unnamed)="CODCr interface Read" ("写入方名称"), element data type=w54) -> (queue out=w55:refnum<queue>)  [unwired: 3 in, 2 out]
    }
  }
  n26 = Not Equal?(x=w12, y=-1) -> (x != y?=w10:bool)
  n27 = Not Equal?(x=w8, y=-1) -> (x != y?=w6:bool)
  n28 = case shown="真" w10 {
    tunnel: [_ w58] -> w28
    tunnel: [_ w57] -> w27
    frame False {
    }
    frame True {
      w57 = T10 {"状态告警区"={"系统时间"=timestamp(0 s since 1904-01-01), "工作状态"=0, "测量模式"=enum."待机", "告警代码"=0, "故障代码"=0, "日志代码"=0, "软件版本"=0, "F0"=0.0, "F1"=0.0, "F2"=0.0, "F3"=0.0, "T"=0.0, "H"=0.0, "id"=0, "flowid"=0, "量程"=0, "总磷控温温度1"=0.0, "营养盐控温温度2"=0.0, "ADC"=0.0}, "平台试剂余量百分比"=0.0, "关键参数"={"测量量程"=0.0, "测量精度"=0.0, "测量间隔"=0.0, "消解温度"=0.0, "消解时长"=0.0, "空白校准时间"=timestamp(0 s since 1904-01-01), "曲线截距"=0.0, "曲线斜率"=0.0, "测量检出限"=0.0, "测量信号值"=0.0, "线性相关系数"=0.0, "二次多项式系数"=0.0, "标样校准时间"=timestamp(0 s since 1904-01-01), "稀释倍数"=0.0, "三项式系数"=0.0, "空白标定系数"=0.0, "量程系数"=0.0, "F0/ORPA"=0.0, "F1/ORPB"=0.0, "F2/ORPK"=0.0, "F3"=0.0, "F4"=0.0, "F5"=0.0, "F6"=0.0, "F7"=0.0, "X0/滴定数"=0.0, "量程"=0.0}, "关键参数改变"=FALSE, "校准信息"={"低标液1浓度"=0.0, "低标液1信号值"=0.0, "低标液1启用"=0, "低标液2浓度"=0.0, "低标液2信号值"=0.0, "低标液2启用"=0, "低标液3浓度"=0.0, "低标液3信号值"=0.0, "低标液3启用"=0, "低标液4浓度"=0.0, "低标液4信号值"=0.0, "低标液4启用"=0, "低标液5浓度"=0.0, "低标液5信号值"=0.0, "低标液5启用"=0, "高标液1浓度"=0.0, "高标液1信号值"=0.0, "高标液1启用"=0, "高标液2浓度"=0.0, "高标液2信号值"=0.0, "高标液2启用"=0, "高标液3浓度"=0.0, "高标液3信号值"=0.0, "高标液3启用"=0, "高标液4浓度"=0.0, "高标液4信号值"=0.0, "高标液4启用"=0, "高标液5浓度"=0.0, "高标液5信号值"=0.0, "高标液5启用"=0}, "校准信息改变"=FALSE}  # 与总磷交互全局
      n29 = Obtain Queue(name (unnamed)="总磷 interface Read" ("写入方名称"), element data type=w57) -> (queue out=w58:refnum<queue>)  [unwired: 3 in, 2 out]
    }
  }
  n30 = case shown="真" w6 {
    tunnel: [_ w61] -> w26
    tunnel: [_ w60] -> w25
    frame False {
    }
    frame True {
      w60 = T11 {"状态告警区"={"系统时间"=timestamp(0 s since 1904-01-01), "工作状态"=0, "测量模式"=enum."待机", "告警代码"=0, "故障代码"=0, "日志代码"=0, "软件版本"=0, "F0"=0.0, "F1"=0.0, "F2"=0.0, "F3"=0.0, "T"=0.0, "H"=0.0, "id"=0, "flowid"=0, "量程"=0, "总磷控温温度1"=0.0, "营养盐控温温度2"=0.0, "ADC"=0.0}, "平台试剂余量百分比"=0.0, "关键参数"={"测量量程"=0.0, "测量精度"=0.0, "测量间隔"=0.0, "消解温度"=0.0, "消解时长"=0.0, "空白校准时间"=timestamp(0 s since 1904-01-01), "曲线截距"=0.0, "曲线斜率"=0.0, "测量检出限"=0.0, "测量信号值"=0.0, "线性相关系数"=0.0, "二次多项式系数"=0.0, "标样校准时间"=timestamp(0 s since 1904-01-01), "稀释倍数"=0.0, "三项式系数"=0.0, "空白标定系数"=0.0, "量程系数"=0.0, "F0/ORPA"=0.0, "F1/ORPB"=0.0, "F2/ORPK"=0.0, "F3"=0.0, "F4"=0.0, "F5"=0.0, "F6"=0.0, "F7"=0.0, "X0/滴定数"=0.0, "量程"=0.0}, "关键参数改变"=FALSE, "校准信息"={"低标液1浓度"=0.0, "低标液1信号值"=0.0, "低标液1启用"=0, "低标液2浓度"=0.0, "低标液2信号值"=0.0, "低标液2启用"=0, "低标液3浓度"=0.0, "低标液3信号值"=0.0, "低标液3启用"=0, "低标液4浓度"=0.0, "低标液4信号值"=0.0, "低标液4启用"=0, "低标液5浓度"=0.0, "低标液5信号值"=0.0, "低标液5启用"=0, "高标液1浓度"=0.0, "高标液1信号值"=0.0, "高标液1启用"=0, "高标液2浓度"=0.0, "高标液2信号值"=0.0, "高标液2启用"=0, "高标液3浓度"=0.0, "高标液3信号值"=0.0, "高标液3启用"=0, "高标液4浓度"=0.0, "高标液4信号值"=0.0, "高标液4启用"=0, "高标液5浓度"=0.0, "高标液5信号值"=0.0, "高标液5启用"=0}, "校准信息改变"=FALSE}  # 与总氮交互全局
      n31 = Obtain Queue(name (unnamed)="总氮 interface Read" ("写入方名称"), element data type=w60) -> (queue out=w61:refnum<queue>)  [unwired: 3 in, 2 out]
    }
  }
  n32 = case shown="真" w1 {
    tunnel: [_ w64] -> w24
    tunnel: [_ w63] -> w23
    frame False {
    }
    frame True {
      w63 = T12 {"状态告警区"={"系统时间"=timestamp(0 s since 1904-01-01), "工作状态"=0, "测量模式"=enum."待机", "告警代码"=0, "故障代码"=0, "日志代码"=0, "软件版本"=0, "F0"=0.0, "F1"=0.0, "F2"=0.0, "F3"=0.0, "T"=0.0, "H"=0.0, "id"=0, "flowid"=0, "量程"=0, "总磷控温温度1"=0.0, "营养盐控温温度2"=0.0, "ADC"=0.0}, "平台试剂余量百分比"=0.0, "关键参数"={"测量量程"=0.0, "测量精度"=0.0, "测量间隔"=0.0, "消解温度"=0.0, "消解时长"=0.0, "空白校准时间"=timestamp(0 s since 1904-01-01), "曲线截距"=0.0, "曲线斜率"=0.0, "测量检出限"=0.0, "测量信号值"=0.0, "线性相关系数"=0.0, "二次多项式系数"=0.0, "标样校准时间"=timestamp(0 s since 1904-01-01), "稀释倍数"=0.0, "三项式系数"=0.0, "空白标定系数"=0.0, "量程系数"=0.0, "F0/ORPA"=0.0, "F1/ORPB"=0.0, "F2/ORPK"=0.0, "F3"=0.0, "F4"=0.0, "F5"=0.0, "F6"=0.0, "F7"=0.0, "X0/滴定数"=0.0, "量程"=0.0}, "关键参数改变"=FALSE, "校准信息"={"低标液1浓度"=0.0, "低标液1信号值"=0.0, "低标液1启用"=0, "低标液2浓度"=0.0, "低标液2信号值"=0.0, "低标液2启用"=0, "低标液3浓度"=0.0, "低标液3信号值"=0.0, "低标液3启用"=0, "低标液4浓度"=0.0, "低标液4信号值"=0.0, "低标液4启用"=0, "低标液5浓度"=0.0, "低标液5信号值"=0.0, "低标液5启用"=0, "高标液1浓度"=0.0, "高标液1信号值"=0.0, "高标液1启用"=0, "高标液2浓度"=0.0, "高标液2信号值"=0.0, "高标液2启用"=0, "高标液3浓度"=0.0, "高标液3信号值"=0.0, "高标液3启用"=0, "高标液4浓度"=0.0, "高标液4信号值"=0.0, "高标液4启用"=0, "高标液5浓度"=0.0, "高标液5信号值"=0.0, "高标液5启用"=0}, "校准信息改变"=FALSE}  # 与氨氮交互全局
      n33 = Obtain Queue(name (unnamed)="氨氮 interface Read" ("写入方名称"), element data type=w63) -> (queue out=w64:refnum<queue>)  [unwired: 3 in, 2 out]
    }
  }
  n34 = Obtain Queue(name (unnamed)=w33, element data type=w38) -> (queue out=w34:refnum<queue>, error out=w37:errorcluster)  [unwired: 3 in, 1 out]
  n35 = Generate Occurrence() -> (w35:refnum<k4>)
  n36 = while {
    tunnel: w34 -> [w68]
    tunnel: w35 -> [w66]
    stop <- w67 stop-if-true
    n37 = event shown="[3] \"启动\": 值改变" {
      selector: _ -> [_ _ _ _ _ _ _ _]
      dyn-events: _ -> [_ _ _ _ _ _ _ _]
      timeout: _ -> [_ _ _ _ _ _ _ _]
      tunnel: w68 -> [_ _ _ w99 w106 w112 w117 w122]
      tunnel: [_ _ _ _ "停止" _ _ _] -> w67
      tunnel: w66 -> [_ _ _ _ w103 _ _ _]
      event Timeout {
        n38 = event-data() -> ()  [unwired: 1 in, 3 out]
      }
      event "启用模块": Value Change {
        n39 = event-data() -> ("NewVal"=w69:bool)  [unwired: 1 in, 5 out]
        n40 = call <vilib>:"Application Directory.vi"() -> ("Application Directory"=w71:path)
        n41 = Build Path(base path=w71, name or relative path="data\\set.ini" ("名称或相对路径")) -> (appended path=w72:path)
        n42 = call <vilib>:"Open Config Data.vi"("configuration file path"=w72) -> ("error out"=w78:errorcluster, "refnum"=w77:T13)  [unwired: 8 in, 1 out]
        n43 = call-poly <vilib>:"Write Key.vi"("section"="总磷总氮", "error in (no error)"=w78, "value"=w69, "key"="模块启用", "refnum"=w77) -> ("error out"=w74:errorcluster, "refnum out"=w70:T13)  [unwired: 4 in, 1 out]
        n44 = call <vilib>:"Close Config Data.vi"("error in (no error)"=w74, "refnum"=w70) -> ()  [unwired: 8 in, 2 out]
      }
      event "VISA Resource": Value Change {
        n45 = event-data() -> ()  [unwired: 1 in, 6 out]
        n46 = call <vilib>:"Application Directory.vi"() -> ("Application Directory"=w81:path)
        n47 = Build Path(base path=w81, name or relative path="data\\set.ini" ("名称或相对路径")) -> (appended path=w82:path)
        n48 = call <vilib>:"Open Config Data.vi"("configuration file path"=w82) -> ("error out"=w88:errorcluster, "refnum"=w87:T13)  [unwired: 8 in, 1 out]
        n49 = call-poly <vilib>:"Write Key.vi"("section"="总磷总氮", "error in (no error)"=w88, "value"="VISA Resource", "key"="串口", "refnum"=w87) -> ("error out"=w84:errorcluster, "refnum out"=w80:T13)  [unwired: 4 in, 1 out]
        n50 = call <vilib>:"Close Config Data.vi"("error in (no error)"=w84, "refnum"=w80) -> ()  [unwired: 8 in, 2 out]
      }
      event "启动": Value Change {
        n51 = event-data() -> ()  [unwired: 1 in, 6 out]
        n52 = case shown="默认" "控制命令" {
          tunnel: "控制命令参数" -> [w101 w102]
          tunnel: [w100 w102] -> w89
          frame Default {
            n53 = call "HexToWord.vi"("数组"=w101) -> ("WORD"=w100:u16[])  [unwired: 10 in]
          }
          frame 13 {
          }
        }
        n54 = Swap Bytes(anything="控制命令") -> (byte swapped=w92:u16)
        n55 = call "控制命令区.vi"("控制命令参数"=w89, "控制命令"=w92) -> ("控制命令"=w95:u16[])  [unwired: 9 in]
        n56 = local read "站号"() -> (w94:u16)
        n57 = Bundle("站号"=w94, "控制命令"=w95) -> (w93:cluster{"站号":u16, "控制命令":u16[]})  [unwired: 1 in]
        n58 = Bundle By Name(cluster=cluster{"命令":string, "data":variant} {"命令"="", "data"=variant} ("元素"), "命令"="启动", "data"=w93) -> (w97:cluster{"命令":string, "data":variant})
        n59 = Enqueue Element(queue=w99, element=w97) -> ()  [unwired: 2 in, 3 out]
      }
      event "停止": Value Change {
        n60 = event-data() -> ()  [unwired: 1 in, 6 out]
        n61 = Set Occurrence(w103) -> ()
        n62 = Flush Queue(queue=w106) -> (queue out=w105:refnum<queue>)  [unwired: 1 in, 2 out]
        n63 = Enqueue Element(queue=w105, element=cluster{"命令":string, "data":variant} {"命令"="shutdown", "data"=variant} ("元素")) -> ()  [unwired: 2 in, 3 out]
      }
      event "读测量数据区": Value Change {
        n64 = event-data() -> ()  [unwired: 1 in, 6 out]
        n65 = Bundle By Name(cluster=cluster{"命令":string, "data":variant} {"命令"="", "data"=variant} ("元素"), "命令"="读测量数据区", "data"="站号") -> (w110:cluster{"命令":string, "data":variant})
        n66 = Enqueue Element(queue=w112, element=w110) -> ()  [unwired: 2 in, 3 out]
      }
      event "读状态告警区": Value Change {
        n67 = event-data() -> ()  [unwired: 1 in, 6 out]
        n68 = local read "站号"() -> (w113:u16)
        n69 = Bundle By Name(cluster=cluster{"命令":string, "data":variant} {"命令"="", "data"=variant} ("元素"), "命令"="读状态告警区", "data"=w113) -> (w115:cluster{"命令":string, "data":variant})
        n70 = Enqueue Element(queue=w117, element=w115) -> ()  [unwired: 2 in, 3 out]
      }
      event "读关键参数区": Value Change {
        n71 = event-data() -> ()  [unwired: 1 in, 6 out]
        n72 = local read "站号"() -> (w118:u16)
        n73 = Bundle By Name(cluster=cluster{"命令":string, "data":variant} {"命令"="", "data"=variant} ("元素"), "命令"="读关键参数区", "data"=w118) -> (w120:cluster{"命令":string, "data":variant})
        n74 = Enqueue Element(queue=w122, element=w120) -> ()  [unwired: 2 in, 3 out]
      }
    }
  }
  n75 = while {
    tunnel: w35 -> [w133]
    tunnel: w34 -> [w129]
    stop <- w130 stop-if-true
    n76 = global read "总磷总氮断电保存全局变量.vi" "MB通信方式选择"() -> (w128:enum16{"串口", "TCP"})
    n77 = Wait on Occurrence(2:w133, 3:10000 ("毫秒超时(-1)")) -> (0:w131:bool)  [unwired: 1 in]
    n78 = Not(x=w131) -> (.not. x?=w130:bool)
    n79 = case shown="\"TCP\"" w128 {
      tunnel: [_ w134] -> w125
      frame "串口", Default {
      }
      frame "TCP" {
        n80 = global read "VAR总磷总氮全局变量.vi" "MB session in"() -> (w136:refnum<class "MB_Master.lvclass">)
        n81 = property class="MB_Master"(reference=w136) -> ("Properties:Session Valid"=w135:bool)  [unwired: 1 in, 2 out]
        n82 = Not(x=w135) -> (.not. x?=w134:bool)
      }
    }
    n83 = First Call?() -> (First Call?: T/F=w127:bool)
    n84 = Or(x=w125, y=w127) -> (x .or. y?=w126:bool)
    n85 = local read "启用"() -> (w123:bool)
    n86 = And(x=w123, y=w126) -> (x .and. y?=w124:bool)
    n87 = case shown="真" w124 {
      tunnel: w129 -> [_ w139]
      frame False {
      }
      frame True {
        n88 = Flush Queue(queue=w139) -> (queue out=w137:refnum<queue>)  [unwired: 1 in, 2 out]
        n89 = Enqueue Element(queue=w137, element=cluster{"命令":string, "data":variant} {"命令"="启用模块", "data"=variant} ("元素")) -> ()  [unwired: 2 in, 3 out]
        n90 = property on="VISA Resource" class="VISAName"("DisabledEnum"=T14."Disabled and Grayed Out" ("禁用")) -> ()  [unwired: 2 in, 2 out]
      }
    }
  }
  n91 = while {
    tunnel: w34 -> [w157]
    tunnel: w37 -> [w156]
    shift-right: [w141] -> _
    shift-left: _ -> [w154]
    tunnel: errorcluster {"status"=FALSE, "code"=0, "source"=""} ("error out") -> [w153]
    tunnel: [w149] -> _
    stop <- w155 stop-if-true
    n92 = Dequeue Element(queue=w157, error in (no error)=w156) -> (queue out=w150:refnum<queue>, element=w151:cluster{"命令":string, "data":variant})  [unwired: 1 in, 2 out]
    n93 = Unbundle By Name(w151) -> ("命令"=w152:string, "data"=w147:variant)
    n94 = case shown="\"读测量数据区\"" w152 {
      tunnel: w147 -> [_ _ _ w195 w206 w223 w244 w293 w313 _]
      tunnel: w150 -> [_ _ _ _ _ _ _ _ _ w326]
      tunnel: [_ _ _ _ _ _ _ _ _ TRUE] -> w155
      tunnel: [w163 w166 w182 w198 w209 w225 w248 w301 w320 w322] -> w141
      tunnel: [w164 w165 w183 w197 w208 w224 w249 w292 w321 w323] -> w149
      tunnel: w154 -> [w163 _ w182 w194 w205 w222 w243 w296 w316 w322]
      tunnel: w153 -> [w164 _ w184 w191 w202 w219 w241 w297 w317 w324]
      tunnel: [_ _ _ w186 w199 w213 w232 w286 w307 _] -> w142
      frame Default {
      }
      frame "启用模块" {
        n95 = global read "总磷总氮断电保存全局变量.vi" "MB通信方式选择"() -> (w167:enum16{"串口", "TCP"})
        n96 = case shown="\"TCP\"" w167 {
          tunnel: [w172 w178] -> w165
          tunnel: [w169 w177] -> w166
          frame "串口", Default {
            n97 = global read "总磷总氮断电保存全局变量.vi" "VISA Resource"() -> (w170:refnum<visa-resource-name>)
            n98 = call <vilib>:"Open Serial Session.vi"("Mode (RTU)"=enum16{"RTU", "ASCII"}."RTU", "Slave ID"=u8 1, "Serial Config"=T16 {"baud rate (bps)"=115200, "stop bits"=10, "parity"=0, "flow control"=0, "timeout"=1000, "retries"=1}, "VISA Resource"=w170) -> ("Error out"=w172:errorcluster, "MB_Serial session"=w169:refnum<class "MB_Master_Serial.lvclass">)  [unwired: 6 in]
          }
          frame "TCP" {
            n99 = global read "总磷总氮断电保存全局变量.vi" "PORT"() -> (w176:string)
            n100 = Decimal String To Number(string=w176) -> (number=w179:i32)  [unwired: 2 in, 1 out]
            n101 = global read "总磷总氮断电保存全局变量.vi" "IP"() -> (w175:string)
            n102 = call <vilib>:"Open TCP Session.vi"("Port (502)"=w179, "IP Address"=w175) -> ("error out"=w178:errorcluster, "MB_TCP session"=w177:refnum<class "MB_Master_TCP.lvclass">)  [unwired: 8 in]
          }
        }
        "启用" <- TRUE
      }
      frame "停用模块" {
        n103 = call-dynamic "Close Session.vi"("error in (no error)"=w184, "MB session in"=w182) -> ("error out"=w180:errorcluster)  [unwired: 9 in]
        n104 = local write "启用"(FALSE ("启用")) -> ()
        n105 = call <vilib>:"Clear Errors.vi"("error in (no error)"=w180) -> ("error out"=w183:errorcluster)  [unwired: 5 in, 1 out]
      }
      frame "启动" {
        n106 = Variant To Data(type=cluster{"站号":u16, "控制命令":u16[]} {"站号"=0, "控制命令"=[]} ("输出簇"), Variant=w195) -> (data=w189:cluster{"站号":u16, "控制命令":u16[]})  [unwired: 1 in, 1 out]
        n107 = Unbundle By Name(w189) -> ("站号"=w186:u16, "控制命令"=w187:u16[])
        n108 = property class="MB_Master"(reference=w194, error in=w191, "Properties:Slave ID"=w186) -> (reference out=w193:refnum<class "MB_Master.lvclass">, error out=w192:errorcluster)
        n109 = Index Array(array=w187) -> (element=w188:u16)  [unwired: 1 in]
        n110 = Swap Bytes(anything=w188) -> (byte swapped=w185:u16)
        n111 = global write "VAR总磷总氮全局变量.vi" "控制命令"(w185) -> ()
        n112 = call <vilib>:"Write Multiple Registers.vi"("error in (no error)"=w192, "values"=w187, "starting address"=u16 4608, "MB session in"=w193) -> ("error out"=w197:errorcluster, "MB session out"=w198:refnum<class "MB_Master.lvclass">)  [unwired: 6 in]
      }
      frame "盲样测试" {
        n113 = Variant To Data(type=u8 0, Variant=w206) -> (data=w199:u8)  [unwired: 1 in, 1 out]
        n114 = property class="MB_Master"(reference=w205, error in=w202, "Properties:Slave ID"=w199) -> (reference out=w204:refnum<class "MB_Master.lvclass">, error out=w203:errorcluster)
        n115 = case shown="默认" w199 {
          tunnel: [u16[] [] ("values") u16[] [33539, 0] ("values") u16[] [23555, 0] ("values")] -> w201
          frame Default {
          }
          frame 1 {
            # "总磷盲样测试命令"
          }
          frame 3 {
            # "氨氮盲样测试"
          }
        }
        n116 = call <vilib>:"Write Multiple Registers.vi"("error in (no error)"=w203, "values"=w201, "starting address"=u16 24592, "MB session in"=w204) -> ("error out"=w208:errorcluster, "MB session out"=w209:refnum<class "MB_Master.lvclass">)  [unwired: 6 in]
      }
      frame "debug" {
        n117 = Variant To Data(type=cluster{"站号":u16, "控制命令":u16[]} {"站号"=0, "控制命令"=[]} ("输出簇"), Variant=w223) -> (data=w217:cluster{"站号":u16, "控制命令":u16[]})  [unwired: 1 in, 1 out]
        n118 = Unbundle By Name(w217) -> ("站号"=w213:u16, "控制命令"=w215:u16[])
        n119 = property class="MB_Master"(reference=w222, error in=w219, "Properties:Slave ID"=w213) -> (reference out=w221:refnum<class "MB_Master.lvclass">, error out=w220:errorcluster)
        n120 = Index Array(array=w215) -> (element=w216:u16)  [unwired: 1 in]
        n121 = global write "VAR总磷总氮全局变量.vi" "控制命令"(w216) -> ()
        n122 = call <vilib>:"Write Multiple Registers.vi"("error in (no error)"=w220, "values"=w215, "starting address"=u16 24594, "MB session in"=w221) -> ("error out"=w224:errorcluster, "MB session out"=w225:refnum<class "MB_Master.lvclass">)  [unwired: 6 in]
      }
      frame "读测量数据区" {
        n123 = Variant To Data(type=u8 1 ("Slave ID"), Variant=w244) -> (data=w232:u8)  [unwired: 1 in, 1 out]
        n124 = property class="MB_Master"(reference=w243, error in=w241, "Properties:Slave ID"=w232) -> (reference out=w242:refnum<class "MB_Master.lvclass">, error out=w240:errorcluster)
        n125 = global read "VAR总磷总氮全局变量.vi" "测量数据区数组"() -> (w237:T8)
        n126 = call "id参数转换.vi"("id"=w232) -> ("数组资源索引"=w231:i32)  [unwired: 9 in, 1 out]
        n127 = call <vilib>:"Read Holding Registers.vi"("error in (no error)"=w240, "quantity"=u16 107, "starting address"=u16 4096, "MB session in"=w242) -> ("error out"=w249:errorcluster, "Registers"=w239:u16[], "MB session out"=w248:refnum<class "MB_Master.lvclass">)  [unwired: 5 in]
        n128 = call "id参数转换.vi"("id"=u16 2) -> ("数组资源索引"=w228:i32)  [unwired: 9 in, 1 out]
        n129 = call "id参数转换.vi"("id"=u16 3) -> ("数组资源索引"=w226:i32)  [unwired: 9 in, 1 out]
        n130 = Index Array(array=w237, index #1=w231, index #2=w228, index #3=w226) -> (element #1=w238:T5, element #2=w233:T5, element #3=w230:T5)
        n131 = call "测量数据区.vi"("数组"=w239) -> ("测量数据区"=w236:T5)  [unwired: 10 in]
        "测量数据区" <- w236
        n132 = global write "VAR总磷总氮全局变量.vi" "测量数据区"(w236) -> ()
        n133 = case shown="1" w232 {
          tunnel: w236 -> [w250 w255 w279 w281 w283]
          tunnel: w239 -> [_ w263 w280 w282 w284]
          tunnel: w238 -> [_ w256 _ _ _]
          tunnel: [w250 w258 w279 w281 w283] -> w235
          tunnel: w233 -> [_ w253 _ _ _]
          tunnel: w230 -> [_ w252 _ _ _]
          frame 0, Default {
          }
          frame 1 {
            n134 = global read "VAR总磷总氮全局变量.vi" "模块名称"() -> (w262:string)
            n135 = Search and Replace String(input string=w262, search string="总磷" ("搜索字符串")) -> (result string=w259:string, offset past replacement=w260:i32)  [unwired: 6 in, 2 out]
            n136 = case shown="-1" w260 {
              tunnel: w259 -> [_ w269]
              tunnel: [_ w266] -> w257
              tunnel: [_ w264] -> w254
              frame -1 {
              }
              frame Default {
                n137 = Search and Replace String(input string=w269, search string="总氮" ("搜索字符串")) -> (offset past replacement=w272:i32)  [unwired: 6 in, 3 out]
                n138 = Search and Replace String(input string=w269, search string="氨氮" ("搜索字符串")) -> (offset past replacement=w267:i32)  [unwired: 6 in, 3 out]
                n139 = Not Equal?(x=w272, y=-1) -> (x != y?=w264:bool)
                n140 = Not Equal?(x=w267, y=-1) -> (x != y?=w265:bool)
                n141 = Or(x=w265, y=w264) -> (x .or. y?=w266:bool)
              }
            }
            n142 = Select(t=w253, s=w254, f=w252) -> (s? t:f=w251:T5)
            n143 = case shown="真" w257 {
              tunnel: [w274 w278] -> w258
              tunnel: w256 -> [_ w277]
              tunnel: w251 -> [_ w276]
              tunnel: w255 -> [w274 w275]
              frame False {
              }
              frame True {
                # "启动总磷总氮时间自动对齐"
                n144 = call "数据时间对齐.vi"("待对齐时间"=w275, "对齐参考时间"=w276, "已对齐时间输入"=w277) -> ("已对齐时间输出"=w278:T5)  [unwired: 8 in]
              }
            }
            "总磷测量数据区" <- w263
          }
          frame 2 {
            "总氮测量数据区" <- w280
          }
          frame 3 {
            "氨氮测量数据区" <- w282
          }
          frame 22 {
            "COD测量数据区" <- w284
          }
        }
        n145 = Replace Array Subset(array=w237, new element=w235, index=w231) -> (w234:T8)
        n146 = global write "VAR总磷总氮全局变量.vi" "测量数据区数组"(w234) -> ()
      }
      frame "读状态告警区" {
        n147 = Variant To Data(type=u8 1 ("Slave ID"), Variant=w293) -> (data=w286:u8)  [unwired: 1 in, 1 out]
        n148 = property class="MB_Master"(reference=w296, error in=w297, "Properties:Slave ID"=w286) -> (reference out=w295:refnum<class "MB_Master.lvclass">, error out=w294:errorcluster)
        n149 = call "id参数转换.vi"("id"=w286) -> ("数组资源索引"=w285:i32)  [unwired: 9 in, 1 out]
        n150 = call <vilib>:"Read Holding Registers.vi"("error in (no error)"=w294, "quantity"=u16 29, "starting address"=u16 4224, "MB session in"=w295) -> ("error out"=w292:errorcluster, "Registers"=w290:u16[], "MB session out"=w301:refnum<class "MB_Master.lvclass">)  [unwired: 5 in]
        n151 = global read "VAR总磷总氮全局变量.vi" "状态告警区数组"() -> (w289:T7)
        n152 = call "状态告警区.vi"("数组"=w290) -> ("状态告警区"=w288:T4)  [unwired: 10 in]
        "状态告警区" <- w288
        n153 = global write "VAR总磷总氮全局变量.vi" "状态告警区"(w288) -> ()
        n154 = Unbundle By Name(w288) -> ("id"=w291:u16)
        n155 = Replace Array Subset(array=w289, new element=w288, index=w285) -> (w287:T7)
        n156 = global write "VAR总磷总氮全局变量.vi" "状态告警区数组"(w287) -> ()
        n157 = case shown="3" w291 {
          tunnel: w288 -> [_ _ _ _ _]
          tunnel: w290 -> [_ w302 w303 w304 w305]
          frame 0, Default {
          }
          frame 1, 131 {
            "总磷状态告警区" <- w302
          }
          frame 2, 76 {
            "总氮状态告警区" <- w303
          }
          frame 3 {
            "氨氮状态告警区" <- w304
          }
          frame 22 {
            "COD状态告警区" <- w305
          }
        }
      }
      frame "读关键参数区" {
        n158 = Variant To Data(type=u8 1 ("Slave ID"), Variant=w313) -> (data=w307:u8)  [unwired: 1 in, 1 out]
        n159 = property class="MB_Master"(reference=w316, error in=w317, "Properties:Slave ID"=w307) -> (reference out=w315:refnum<class "MB_Master.lvclass">, error out=w314:errorcluster)
        n160 = call "id参数转换.vi"("id"=w307) -> ("数组资源索引"=w306:i32)  [unwired: 9 in, 1 out]
        n161 = call <vilib>:"Read Holding Registers.vi"("error in (no error)"=w314, "quantity"=u16 19, "starting address"=u16 4256, "MB session in"=w315) -> ("error out"=w321:errorcluster, "Registers"=w311:u16[], "MB session out"=w320:refnum<class "MB_Master.lvclass">)  [unwired: 5 in]
        n162 = global read "VAR总磷总氮全局变量.vi" "关键参数区数组"() -> (w310:T6)
        n163 = call "关键参数区.vi"("数组"=w311) -> ("关键参数区"=w309:T3)  [unwired: 10 in]
        "关键参数区" <- w309
        n164 = global write "VAR总磷总氮全局变量.vi" "关键参数区"(w309) -> ()
        n165 = Replace Array Subset(array=w310, new element=w309, index=w306) -> (w308:T6)
        n166 = global write "VAR总磷总氮全局变量.vi" "关键参数区数组"(w308) -> ()
      }
      frame "shutdown" {
        n167 = call-dynamic "Close Session.vi"("error in (no error)"=w324, "MB session in"=w322) -> ("error out"=w323:errorcluster)  [unwired: 9 in]
        n168 = Flush Queue(queue=w326) -> (queue out=w325:refnum<queue>)  [unwired: 1 in, 2 out]
        n169 = Release Queue(queue=w325) -> ()  [unwired: 2 in, 3 out]
      }
    }
    n170 = global write "VAR总磷总氮全局变量.vi" "MB session in"(w141) -> ()
    n171 = Unbundle By Name(w149) -> ("status"=w145:bool)
    n172 = Not(x=w145) -> (.not. x?=w148:bool)
    "status" <- w148
    n173 = call <vilib>:"Boolean Crossing PtByPt.vi"("direction"=enum16{"either", "false-true", "true-false"}."false-true", "input"=w145) -> ("crossing"=w144:bool)  [unwired: 1 in]
    n174 = call "id参数转换.vi"("id"=w142) -> ("table输出"=w146:string)  [unwired: 9 in, 1 out]
    n175 = case shown="真" w144 {
      tunnel: w146 -> [_ w162]
      frame False {
      }
      frame True {
        n176 = Get Date/Time In Seconds() -> (seconds since 1Jan1904=w161:timestamp)
        n177 = Bundle By Name(cluster=T15 {"时间"=timestamp(0 s since 1904-01-01), "参数"="", "报警信息"="", "备注"="", "code"=0, "platform_alarm_code"="", "报警标识"=enum."产生"} ("data in"), "时间"=w161, "参数"=w162, "报警信息"="通讯告警" ("日志信息")) -> (w158:T15)
        n178 = call "总磷总氮报警信息.vi"("data in"=w158) -> ()  [unwired: 10 in, 1 out]
      }
    }
    n179 = global write "VAR总磷总氮全局变量.vi" "通讯状态"(w148) -> ()
  }
  n180 = while {
    tunnel: w32 -> [w337]
    tunnel: w31 -> [w336]
    tunnel: w30 -> [w335]
    tunnel: w29 -> [w334]
    tunnel: w28 -> [w333]
    tunnel: w27 -> [w332]
    tunnel: w26 -> [w331]
    tunnel: w25 -> [w330]
    tunnel: w24 -> [w329]
    tunnel: w23 -> [w328]
    stop <- FALSE stop-if-true
    n181 = global read "model config var.vi" "启动队列名称"() -> (w340:cluster{"String":string, "Value":u16}[])
    n182 = Wait (ms)(milliseconds to wait=u32 1000 ("等待时间（毫秒）")) -> ()  [unwired: 1 out]
    n183 = for {
      tunnel: w340 -> [w352] mode=indexing
      tunnel: w337 -> [w350]
      tunnel: w336 -> [w349]
      tunnel: w335 -> [w348]
      tunnel: w334 -> [w347]
      tunnel: w333 -> [w346]
      tunnel: w332 -> [w345]
      tunnel: w331 -> [w344]
      tunnel: w330 -> [w343]
      tunnel: w329 -> [w342]
      tunnel: w328 -> [w341]
      n184 = Unbundle By Name(w352) -> ("Value"=w351:u16)
      n185 = case shown="1" w351 {
        tunnel: w350 -> [_ _ _ _ w430 _]
        tunnel: w349 -> [_ _ _ _ w429 _]
        tunnel: w348 -> [_ _ _ w411 _ _]
        tunnel: w347 -> [_ _ _ w410 _ _]
        tunnel: w346 -> [w354 _ _ _ _ _]
        tunnel: w345 -> [w353 _ _ _ _ _]
        tunnel: w344 -> [_ w373 _ _ _ _]
        tunnel: w343 -> [_ w372 _ _ _ _]
        tunnel: w342 -> [_ _ w392 _ _ _]
        tunnel: w341 -> [_ _ w391 _ _ _]
        frame 1 {
          n186 = Get Queue Status(queue=w354) -> (queue out=w357:refnum<queue>, # elements in queue=w356:i32)  [unwired: 2 in, 6 out]
          n187 = Equal To 0?(x=w356) -> (x = 0?=w355:bool)
          n188 = case shown="真" w355 {
            tunnel: w353 -> [_ w368]
            tunnel: w357 -> [_ w369]
            frame False {
            }
            frame True {
              w359 = u16 1 items=["总磷"=1, "总氮"=2, "氨氮"=3, "磷酸盐"=4, "硝氮"=5, "亚硝氮"=6, "硅酸盐"=7, "硫化物"=8, "CODCr"=22]
              n189 = Unbundle By Name(w368) -> ("关键参数"=w366:T17)
              n190 = global read "VAR总磷总氮全局变量.vi" "总磷关键参数"() -> (w367:T18)
              n191 = global read "VAR总磷总氮全局变量.vi" "状态告警区数组"() -> (w361:T7)
              n192 = global read "VAR总磷总氮全局变量.vi" "平台试剂余量百分比"() -> (w371:sgl)
              n193 = call "id参数转换.vi"("id"=w359) -> ("数组资源索引"=w360:i32)  [unwired: 9 in, 1 out]
              n194 = call "转换关键参数(子VI).vi"("参数"=w359, "总磷关键参数"=w367, "关键参数输入"=w366) -> ("关键参数输出"=w365:T17)  [unwired: 8 in]
              n195 = global read "VAR总磷总氮全局变量.vi" "总磷关键参数改变"() -> (w364:bool)
              n196 = global read "VAR总磷总氮全局变量.vi" "总磷校准信息改变"() -> (w362:bool)
              n197 = global read "VAR总磷总氮全局变量.vi" "总磷校准信息"() -> (w363:T19)
              n198 = Index Array(array=w361, index=w360) -> (element=w358:T4)
              n199 = Bundle By Name(cluster=w368, "状态告警区"=w358, "平台试剂余量百分比"=w371, "关键参数"=w365, "关键参数改变"=w364, "校准信息"=w363, "校准信息改变"=w362) -> (w370:T10)
              n200 = Enqueue Element(queue=w369, element=w370) -> ()  [unwired: 2 in, 3 out]
            }
          }
        }
        frame 2 {
          n201 = Get Queue Status(queue=w373) -> (queue out=w376:refnum<queue>, # elements in queue=w375:i32)  [unwired: 2 in, 6 out]
          n202 = Equal To 0?(x=w375) -> (x = 0?=w374:bool)
          n203 = case shown="真" w374 {
            tunnel: w376 -> [_ w388]
            tunnel: w372 -> [_ w386]
            frame False {
            }
            frame True {
              w378 = u16 2 items=["总磷"=1, "总氮"=2, "氨氮"=3, "磷酸盐"=4, "硝氮"=5, "亚硝氮"=6, "硅酸盐"=7, "硫化物"=8, "CODCr"=22]
              n204 = Unbundle By Name(w386) -> ("关键参数"=w385:T17)
              n205 = global read "VAR总磷总氮全局变量.vi" "总氮关键参数"() -> (w387:T18)
              n206 = global read "VAR总磷总氮全局变量.vi" "状态告警区数组"() -> (w379:T7)
              n207 = global read "VAR总磷总氮全局变量.vi" "平台试剂余量百分比"() -> (w390:sgl)
              n208 = call "id参数转换.vi"("id"=w378) -> ("数组资源索引"=w380:i32)  [unwired: 9 in, 1 out]
              n209 = call "转换关键参数(子VI).vi"("参数"=w378, "总磷关键参数"=w387, "关键参数输入"=w385) -> ("关键参数输出"=w384:T17)  [unwired: 8 in]
              n210 = global read "VAR总磷总氮全局变量.vi" "总氮关键参数改变"() -> (w383:bool)
              n211 = global read "VAR总磷总氮全局变量.vi" "总氮校准信息改变"() -> (w381:bool)
              n212 = global read "VAR总磷总氮全局变量.vi" "总氮校准信息"() -> (w382:T19)
              n213 = Index Array(array=w379, index=w380) -> (element=w377:T4)
              n214 = Bundle By Name(cluster=w386, "状态告警区"=w377, "平台试剂余量百分比"=w390, "关键参数"=w384, "关键参数改变"=w383, "校准信息"=w382, "校准信息改变"=w381) -> (w389:T11)
              n215 = Enqueue Element(queue=w388, element=w389) -> ()  [unwired: 2 in, 3 out]
            }
          }
        }
        frame 3 {
          (unwired) FALSE
          n216 = Get Queue Status(queue=w392) -> (queue out=w394:refnum<queue>, # elements in queue=w395:i32)  [unwired: 2 in, 6 out]
          n217 = Equal To 0?(x=w395) -> (x = 0?=w393:bool)
          n218 = case shown="真" w393 {
            tunnel: w394 -> [_ w407]
            tunnel: w391 -> [_ w406]
            frame False {
            }
            frame True {
              w397 = u16 3 items=["总磷"=1, "总氮"=2, "氨氮"=3, "磷酸盐"=4, "硝氮"=5, "亚硝氮"=6, "硅酸盐"=7, "硫化物"=8, "CODCr"=22]
              n219 = Unbundle By Name(w406) -> ("关键参数"=w405:T17)
              n220 = global read "VAR总磷总氮全局变量.vi" "氨氮关键参数"() -> (w403:T18)
              n221 = global read "VAR总磷总氮全局变量.vi" "状态告警区数组"() -> (w398:T7)
              n222 = global read "VAR总磷总氮全局变量.vi" "平台试剂余量百分比"() -> (w409:sgl)
              n223 = call "id参数转换.vi"("id"=w397) -> ("数组资源索引"=w399:i32)  [unwired: 9 in, 1 out]
              n224 = call "转换关键参数(子VI).vi"("参数"=w397, "总磷关键参数"=w403, "关键参数输入"=w405) -> ("关键参数输出"=w404:T17)  [unwired: 8 in]
              n225 = global read "VAR总磷总氮全局变量.vi" "氨氮关键参数改变"() -> (w402:bool)
              n226 = global read "VAR总磷总氮全局变量.vi" "氨氮校准信息改变"() -> (w400:bool)
              n227 = global read "VAR总磷总氮全局变量.vi" "氨氮校准信息"() -> (w401:T19)
              n228 = Index Array(array=w398, index=w399) -> (element=w396:T4)
              n229 = Bundle By Name(cluster=w406, "状态告警区"=w396, "平台试剂余量百分比"=w409, "关键参数"=w404, "关键参数改变"=w402, "校准信息"=w401, "校准信息改变"=w400) -> (w408:T12)
              n230 = Enqueue Element(queue=w407, element=w408) -> ()  [unwired: 2 in, 3 out]
            }
          }
        }
        frame 22 {
          n231 = Get Queue Status(queue=w411) -> (queue out=w413:refnum<queue>, # elements in queue=w414:i32)  [unwired: 2 in, 6 out]
          n232 = Equal To 0?(x=w414) -> (x = 0?=w412:bool)
          n233 = case shown="真" w412 {
            tunnel: w413 -> [_ w426]
            tunnel: w410 -> [_ w425]
            frame False {
            }
            frame True {
              w416 = u16 22 items=["总磷"=1, "总氮"=2, "氨氮"=3, "磷酸盐"=4, "硝氮"=5, "亚硝氮"=6, "硅酸盐"=7, "硫化物"=8, "CODCr"=22]
              n234 = Unbundle By Name(w425) -> ("关键参数"=w424:T17)
              n235 = global read "VAR总磷总氮全局变量.vi" "CODcr关键参数"() -> (w423:T18)
              n236 = global read "VAR总磷总氮全局变量.vi" "状态告警区数组"() -> (w417:T7)
              n237 = global read "VAR总磷总氮全局变量.vi" "CODCr关键参数改变"() -> (w421:bool)
              n238 = global read "VAR总磷总氮全局变量.vi" "CODCr校准信息改变"() -> (w419:bool)
              n239 = global read "VAR总磷总氮全局变量.vi" "平台试剂余量百分比"() -> (w428:sgl)
              n240 = call "id参数转换.vi"("id"=w416) -> ("数组资源索引"=w418:i32)  [unwired: 9 in, 1 out]
              n241 = call "转换关键参数(子VI).vi"("参数"=w416, "总磷关键参数"=w423, "关键参数输入"=w424) -> ("关键参数输出"=w422:T17)  [unwired: 8 in]
              n242 = global read "VAR总磷总氮全局变量.vi" "CODCr校准信息"() -> (w420:T19)
              n243 = Index Array(array=w417, index=w418) -> (element=w415:T4)
              n244 = Bundle By Name(cluster=w425, "状态告警区"=w415, "平台试剂余量百分比"=w428, "关键参数"=w422, "关键参数改变"=w421, "校准信息"=w420, "校准信息改变"=w419) -> (w427:T9)
              n245 = Enqueue Element(queue=w426, element=w427) -> ()  [unwired: 2 in, 3 out]
            }
          }
        }
        frame 21 {
          (unwired) FALSE
          n246 = Get Queue Status(queue=w430) -> (queue out=w432:refnum<queue>, # elements in queue=w433:i32)  [unwired: 2 in, 6 out]
          n247 = Equal To 0?(x=w433) -> (x = 0?=w431:bool)
          n248 = case shown="真" w431 {
            tunnel: w432 -> [_ w445]
            tunnel: w429 -> [_ w444]
            frame False {
            }
            frame True {
              w435 = u16 21 items=["总磷"=1, "总氮"=2, "氨氮"=3, "磷酸盐"=4, "硝氮"=5, "亚硝氮"=6, "硅酸盐"=7, "硫化物"=8, "CODMn"=21, "CODCr"=22, "氟化物"=50]
              n249 = Unbundle By Name(w444) -> ("关键参数"=w443:T17)
              n250 = global read "VAR总磷总氮全局变量.vi" "CODMn关键参数"() -> (w442:T18)
              n251 = global read "VAR总磷总氮全局变量.vi" "状态告警区数组"() -> (w436:T7)
              n252 = global read "VAR总磷总氮全局变量.vi" "CODmn关键参数改变"() -> (w440:bool)
              n253 = global read "VAR总磷总氮全局变量.vi" "CODMn校准信息改变"() -> (w438:bool)
              n254 = global read "VAR总磷总氮全局变量.vi" "平台试剂余量百分比"() -> (w447:sgl)
              n255 = call "id参数转换.vi"("id"=w435) -> ("数组资源索引"=w437:i32)  [unwired: 9 in, 1 out]
              n256 = call "转换关键参数(子VI).vi"("参数"=w435, "总磷关键参数"=w442, "关键参数输入"=w443) -> ("关键参数输出"=w441:T17)  [unwired: 8 in]
              n257 = global read "VAR总磷总氮全局变量.vi" "CODMn校准信息"() -> (w439:T19)
              n258 = Index Array(array=w436, index=w437) -> (element=w434:T4)
              n259 = Bundle By Name(cluster=w444, "状态告警区"=w434, "平台试剂余量百分比"=w447, "关键参数"=w441, "关键参数改变"=w440, "校准信息"=w439, "校准信息改变"=w438) -> (w446:T9)
              n260 = Enqueue Element(queue=w445, element=w446) -> ()  [unwired: 2 in, 3 out]
            }
          }
        }
        frame Default {
        }
      }
    }
  }
